vi "Daq.Gui.vi"() -> ()   [LabVIEW 2016]
uses:
  Daq.Gui.Action.ctl
  Drivers/V7310/V7310.Data.Status.State.ctl
  Drivers/V7310/LowLevel/V7310.LaserStatus.ctl
  Drivers/FestoCPX/Station/FestoCPX.Station.ProdPresentGUI.ctl
  Drivers/FestoCPX/Station/FestoCPX.Station.RevolverID.ctl
  Drivers/V7310/LowLevel/V7310.Job.Sets.ctl
  tools/Translator/Translator.Message.ctl
  Drivers/V7310/LowLevel/V7310.Job.Data.ctl
  Station/Station.ValvePosition.ctl
  Station/Station.ProductSlot.ctl
  Drivers/FestoCPX/Station/FestoCPX.Station.ProdArmPosition.ctl
  <vilib>/Utility/miscctls.llb/LVRowAndColumnTypeDef.ctl
  Drivers/FestoCPX/FestoCPX.DO.Data.Fglb.Action.ctl
  tools/CitTemplate/citTemplate.errData.ctl
  tools/EventLog/EventLog.EventSource.ctl
  Station/Station.ProductSuctionGripper.Type.ctl
  tools/Translator/Translator.FormatMessage.vi
  tools/Config/Config.Global.vi
  Global/ApplicationGlobal.vi
  tools/Translator/Translator.Global.vi
  Drivers/FestoCPX/FestoCPX.Global.vi
  Drivers/V7310/LowLevel/V7310.Global.vi
  Sequence/Sequence.Global.vi
  Station/Station.Global.vi
panel:
  out "Run.PeriphsHider 2":bool
  out "Run.PeriphsHider":bool
  out "_loop":i32(ring)=4
  in  "MainTab":enum32{"TABLE", "LASER"}(tab)
  out "ForkID":u8 caption="PopID"
  in  "Btn10":bool caption="Produkt"
  in  "Btn09":bool caption="Blokada"
  in  "Btn07":bool caption="Arm"
  in  "Btn08":bool caption="Arm"
  in  "Btn06":bool caption="Ramię"
  in  "Btn03":bool caption="Table"
  out "RevolverID":T1 caption="MagID"
  in  "Btn17":bool caption="Sucker Slot L B"
  in  "Btn16":bool caption="Sucker Slot L A"
  in  "Btn18":bool caption="Sucker Slot T A"
  in  "Btn19":bool caption="Sucker Slot T B"
  in  "Btn20":bool caption="Sucker Slot R A"
  in  "Btn21":bool caption="Sucker Slot R B"
  in  "Btn22":bool caption="Sucker Slot B A"
  in  "Btn23":bool caption="Sucker Slot B B"
  in  "Btn04":bool caption="Lift"
  in  "Btn15":bool caption="Koniec"
  in  "Btn14":bool caption="Final"
  in  "Btn05":bool caption="Stół"
  out "ProdPresent":T2
  in  "Laser.PrintB":bool
  in  "Laser.Job.SetsB":T3 caption="B"
  out "Laser.JobInUse":string caption="Wybrany program"
  out "Laser.Job.VarDef":string[](array[string]) caption="Zmienne"
  out "EmgFrontDoorSecured":bool caption="Bezp. Blokada Drzwi"
  out "EmgSideDoor":bool caption="Bezp. Drzwi Bok"
  out "EmgFrontDoor":bool caption="Bezp. Drzwi Front"
  out "EmgButton":bool caption="Bezp. Wyłącznik"
  in  "Btn01":bool caption="Bezp."
  in  "Btn02":bool caption="Blokada\nDrzwi"
  in  "Laser.Job.SetsA":T3 caption="A"
  out "Laser.LaserStatusRaw":string caption="Status"
  out "Laser.TS":timestamp caption="Czas"
  out "Laser.Status":T4 caption="Status"
  out "Laser.State":T5=enum."Init" caption="Stan"
  in  "Btn11":bool caption="Interlock"
  in  "Btn13":bool caption="Odsysacz\noparów"
  in  "Btn12":bool caption="Wyzwolenie"
  in  "Job.Variables":string[](array[string]) caption="Wartości"
  out "AirPressureInside":bool caption="Ciśnienie wewnątrz"
  out "AirPressure":bool caption="Ciśnienie zasilania"
  in  "Btn00":bool caption="Powietrze"
  in  "ScanOrder":bool
  in  "ScanProduct":bool
  in  "Laser.PrintA":bool
  in  "DO.Manual":bool caption="Control"
  in  "DO.Buttons":bool[](array[boolean])
  out "DO":i32(listbox)
  out "DI":i32(listbox)=-1
  out "ButtRefs":refnum<vi>[](array[refnum])
  out "delay":u32
  out "exit":bool
  out "Panel":refnum<vi>
  out "action":T6=enum."--- Daq.Gui ---"
  in  "_align":bool
  # "RAW DATA"
  # "TABLE"
  # "EMERGENCY CIRCUIT"
  # "AIR PRESSURE"
  # "SCANNER"
  # "LASER"
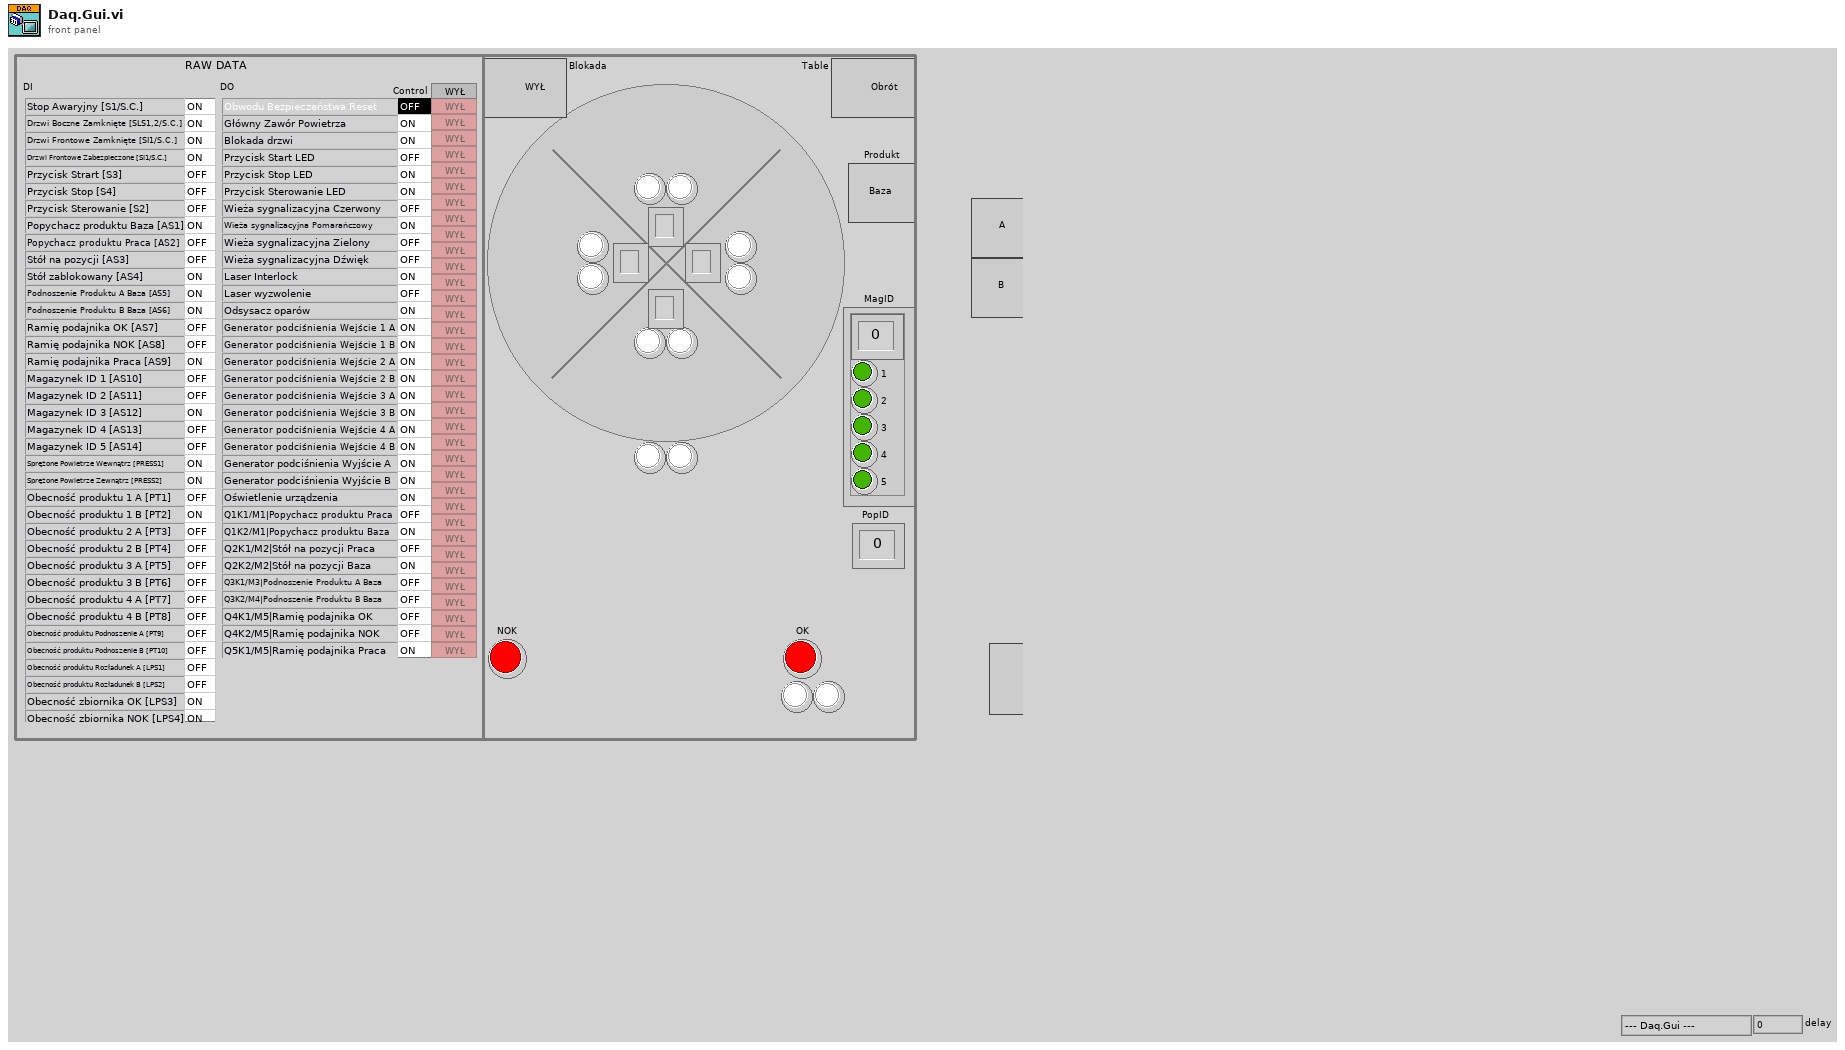
[diagram p1: front panel]
types:
  T1 = typedef "FestoCPX.Station.RevolverID.ctl" = cluster{"ID":u8, "1":bool, "2":bool, "3":bool, "4":bool, "5":bool}
  T2 = typedef "FestoCPX.Station.ProdPresentGUI.ctl" = cluster{"ProdPresentSlotRightA":bool, "ProdPresentSlotRightB":bool, "ProdPresentSlotTopA":bool, "ProdPresentSlotTopB":bool, "ProdPresentSlotLeftA":bool, "ProdPresentSlotLeftB":bool, "ProdPresentSlotBottomA":bool, "ProdPresentSlotBottomB":bool, "SlotNoRight":u8, "SlotNoTop":u8, "SlotNoLeft":u8, "SlotNoBottom":u8, "ProdFinalA":bool, "ProdFinalB":bool, "ProdFinalA 2":bool, "ProdFinalB 2":bool, "ProdContainerOK":bool, "ProdContainerNOK":bool}
  T3 = typedef "V7310.Job.Sets.ctl" = cluster{"X":dbl, "Y":dbl, "Angle":dbl}
  T4 = typedef "V7310.LaserStatus.ctl" = enum16{"-", "FatalError", "Initialize", "KeySwitchOpen", "TimeoutInterlock", "InterlockOpen", "StartUp", "ShutterlockOpen", "Standby", "Ready", "PrepareForMarking", "WaitForTrigger", "Marking"}
  T5 = typedef "V7310.Data.Status.State.ctl" = enum16{"First", "Init", "Msg", "Error", "Abort", "Idle", "Run"}
  T6 = typedef "Daq.Gui.Action.ctl" = enum32{"idle", "constructor", "destructor", "--- Daq.Gui ---", "Open", "Update.IO", "Update.Buttons"}
  T7 = enum8{"Enabled", "Disabled", "Disabled and Grayed Out"}
  T8 = typedef "V7310.Job.Data.ctl" = cluster{"Vars":string[], "Sets":T3}
  T9 = typedef "Translator.Message.ctl" = enum16{"-", "Event confirmed", "Log out", "Log in", "Shutdown", "Cancel", "Start", "Begin time", "End time", "Duration", "Service Mode", "Ignore Results", "Serial Format", "On", "Off", "OK", "NOK", "NOK %s", "Home", "Work", "Close", "Open", "In progress...", "Missing", "Empty", "Hardware failure", "Initial", "Default", "Total", "Out of range", "Free disk space is below 1GB - contact technician", "Error %d >> %s", "Error %d >> %s >> %s", "Msg %d >> %s", "Laser msg %d %s", "Laser cmd error %s %d", "Laser cmd failed %s", "Laser cmd warning %s", "Laser disconnected", "Laser status %s", "Laser already started", "Laser job unkonwn %s", "Laser job missing %s", "Laser job select failure %s", "Unable to start laser printing (%s)", "Unable to stop laser printing (%s)", "Laser marking aborted", "Laser marking timeout", "Unable to reset Laser Interlock (%s)", "Unable to trigger Laser. Laser not ready (%s)", "Laser job '%s' coordinates not configured", "Starting %s", "Quitting %s", "Configured", "Initializing", "Quitting", "Loading", "Loaded %d results", "Loaded %d events", "Running", "Stopped", "Summary", "Laser", "Do you want to continue?", "Do you want to delete the configuration?", "The configuration is being used by an order. Unable to delete!", "Press confirm button", "Station is not based. Do you want to exit?", "Station requires changeover. Do you want to run the test?", "Test options are not set as default. Do you want to continue?", "Formatting of WabcoNo is disabled. Do you want to continue?", "Product not detected. Do you want to continue?", "Product scan failed. Do you want to continue?", "Calibration", "Log out?", "System", "All", "IDLE", "Translating...%s", "Not found", "Alarm %s", "Run", "Skip", "Abort", "Repeat", "Please wait...", "Database disconnected", "Database disconnected - changeover disabled!", "Login to database successful", "Login to database failed: %d; %s", "Unable to check the product status of reference %d - database disconnected", "Unable to set the product status of reference %d - database disconnected", "Variant file backup %s", "Read variant (%s)", "Result", "Station armed!", "Station requires changeover!", "Select reference number...", "EMERGENCY BUTTON - press Control button", "EMERGENCY DOOR - press Control button", "Resetting Emergency...", "Unable to reset safety circuit - Emergency Button pressed", "Unable to reset safety circuit - Emergency Side Door open", "Station not based", "Station based", "Station not empty", "Station basing...", "No order", "Press Start to begin new order", "Scanning new order", "Order NOK. Correct or scan again", "Order OK. Press Accept", "Order ready", "Revolver incorrect", "Fork incorrect", "Revolver missing", "Revolver empty", "Container missing", "Offline results", "Offline statistics", "Updating statistics %.1f %%", "DMC Configurator", "Door open", "Close the front door", "Press start button", "Done. Open the front door", "Running...", "Running...%.1f %%", "Pause %s", "Pause %s. NOK container missing", "Pause %s. OK container missing", "Pause %s. Revolver empty", "Pause %s. Revolver missing", "Pause %s. Revolver incorrect", "Pause %s. Fork missing", "Pause %s. Fork incorrect", "Pause %s. Too many failures", "Pause %s. Unloading failure", "Pause %s. One slot is not working", "Pause %s. Part order is done. Empty OK container", "Pause %s. Unable to move product to slot", "Pause %s. Unable to move back product pusher", "Pause %s. Unable to lift product", "Pause %s. Unable to move back product lifter", "Pause %s. Unable to move product arm to Work", "Pause %s. Unable to move product arm to NOK", "Pause %s. Unable to move product arm to OK", "Pause %s. Unable to unsuck the NOK product", "Pause %s. Unable to drop the NOK product", "Pause %s. Product OK missing", "Pause %s. Unable to unsuck the OK product", "Pause %s. Unable to drop the OK product", "Stopping...", "File '%s' is missing", "File '%s' is broken", "File '%s' is running", "Log file started (%s)", "Log file ended (%s)", "Log file stopped (%s)", "Log file ignored (%s)", "Log file exported (%s)", "Log file export failed (%s)", "Wrong serial number in log file", "Wrong reference number in log file", "Test steps are missing", "%s = %.3f", "Process param '%s' not found in DB", "Process param '%s' wrong order", "Process param '%s' value %.3f out of limits (%.3f; %.3f)", "Step%d param '%s' not found in DB", "Step%d param '%s' wrong order", "Step%d param '%s' value %.3f out of limits (%.3f; %.3f)", "Step%d EV '%s' not found in DB", "Step%d EV '%s' wrong order", "\"%s\" not found in DB", "\"%s\" wrong order", "\"%s\" value %.3f out of limits (%.3f; %.3f)", "\"%s\" not found in software", "Process init (%s)", "Process started", "Process restarted", "Process run", "Process done", "Process done - remove OK container", "Process aborted", "Process aborted at work", "Process aborted at home", "Process error", "Process error at home", "Process error at work", "Process close", "Process pause", "Process continue", "Process door open", "Process door close", "Process pause at slot %s due to %s", "Select plate from the order to process", "Do you want to start the process?", "Do you want to continue the process?", "There is unfinished order. Do you want to put the new order?", "Product %s %d OK", "Product %s %d NOK", "Unable to unload the slot %s. Product missing in the slot", "Unable to unload the slot %s. Product already in the arm", "Unable to accept the product as OK. Product missing in slot %s", "Unable to accept the product as OK. Product could not drop into the container at slot %s", "Unable to accept the product as NOK. Product could not drop into the container at slot %s", "Scan failed. Error %s", "Scan failed. Scanner disconnected", "Scan failed. Wrong Wabco number %d, limit (%d,%d)", "Scan failed. Wrong serial number %d, limit (%d,%d)", "Scan failed. Wrong date %d, limit (%d,%d)", "Scan failed. Wrong product wabco number %d (expected %d)", "Scan failed. Wrong product serial number %d (expected > 0)", "Scan OK %s", "Scan failed. Unable to determine table position (%s)", "Scan failed. Timeout", "Tune failed. Scanner disconnected", "Tune failed. Timeout", "%s = %d", "%s = %d->%d", "Unable to set %s = %.2f - Air Pressure Inside off", "Unable to set digital output '%s' = %d", "Unable to activate air pressure inside - timeout", "Unable to activate air pressure inside - aborted", "Unable to switch on Air Main Valve - Air Pressure Inlet off", "Unable to switch on Air Main Valve - Door open", "Unable to switch off Air Main Valve - timeout", "Unable to switch off Air Main Valve - aborted", "Unable to rotate Table - timeout", "Unable to rotate Table - aborted", "Unable to rotate Table - Product Move not in Home position", "Unable to rotate Table - Air Pressure Inside off", "Unable to rotate Table - Product Lift A not in Home position", "Unable to rotate Table - Product Lift B not in Home position", "Unable to rotate Table - unlock before movement timeout", "Unable to rotate Table - lock after movement timeout", "Unable to move Table Lock to %s position - timeout", "Unable to move Table Lock to %s position - aborted", "Unable to move Table Lock to %s position - Air Pressure Inside off", "Unable to move Table Lock to %s position - Table not in position", "Unable to move Product Lift A to %s position - timeout", "Unable to move Product Lift B to %s position - timeout", "Unable to move Product Lift A to %s position - aborted", "Unable to move Product Lift B to %s position - aborted", "Unable to move Product Lift A to %s position - Air Pressure Inside off", "Unable to move Product Lift B to %s position - Air Pressure Inside off", "Unable to move Product Lift A to %s position - Table not locked", "Unable to move Product Lift B to %s position - Table not locked", "Unable to move Product Lift A to %s position - Product Arm not in Work position", "Unable to move Product Lift B to %s position - Product Arm not in Work position", "Unable to set Product Suction Gripper %s to %s - timeout", "Unable to set Product Suction Gripper %s to %s - aborted", "Unable to set Product Suction Gripper %s to %s - Air Pressure Inside off", "Unable to set Product Suction Gripper %s to %s - Table slot unkown", "Unable to move Product Arm to %s position - timeout", "Unable to move Product Arm to %s position - aborted", "Unable to move Product Arm to %s position - Air Pressure Inside off", "Unable to move Product Arm to %s position - Product Lift A not in Home position", "Unable to move Product Arm to %s position - Product Lift B not in Home position", "Unable to move Product to %s position - timeout", "Unable to move Product to %s position - aborted", "Unable to move Product to %s position - Air Pressure Inside off", "Unable to move Product to %s position - Table not in position"}
  T10 = typedef "Station.ValvePosition.ctl" = enum16{"Home", "Work"}
  T11 = typedef "Station.ProductSlot.ctl" = enum8{"A", "B"}
  T12 = typedef "FestoCPX.Station.ProdArmPosition.ctl" = enum16{"Work", "OK", "NOK"}
  T13 = typedef "LVRowAndColumnTypeDef.ctl" = cluster{"Row":i32, "Column":i32}
  T14 = typedef "FestoCPX.DO.Data.Fglb.Action.ctl" = enum16{"init", "set", "get", "check", "select", "reset"}
  T15 = typedef "EventLog.EventSource.ctl" = enum16{"All", "Gui", "Ref", "File", "Arch", "Seq", "CPX", "DB", "Laser", "Scan.P", "Scan.O"}
  T16 = typedef "citTemplate.errData.ctl" = cluster{"ts":timestamp, "src":T15, "instance":i32, "action":string, "error":errorcluster, "unconfirmed":bool}
  T17 = typedef "Station.ProductSuctionGripper.Type.ctl" = enum8{"Final A", "Final B", "Slot 1 A", "Slot 1 B", "Slot 2 A", "Slot 2 B", "Slot 3 A", "Slot 3 B", "Slot 4 A", "Slot 4 B"}
  T18 = typedef "citTemplate.notifierHandle.ctl" = refnum<notifier>
  T19 = enum32{"Invalid", "Standard", "Closed", "Hidden", "Minimized", "Maximized"}
  T20 = typedef "LVPositionTypeDef.ctl" = cluster{"Left":i32, "Top":i32}
  T21 = typedef "FestoCPX.Data.Sets.ctl" = cluster{"IP":string, "Timeout_ms":i32, "ReconnectPeriod_s":i32, "Config.DI":T22[], "Config.DO":T24[]}
  T22 = typedef "FestoCPX.DI.Sets.ctl" = cluster{"Name":string, "Channel":T23, "Negate":bool}
  T23 = typedef "FestoCPX.DI.ctl" = enum16{"0.0", "0.1", "0.2", "0.3", "0.4", "0.5", "0.6", "0.7", "1.0", "1.1", "1.2", "1.3", "1.4", "1.5", "1.6", "1.7", "2.0", "2.1", "2.2", "2.3", "2.4", "2.5", "2.6", "2.7", "3.0", "3.1", "3.2", "3.3", "3.4", "3.5", "3.6", "3.7", "4.0", "4.1", "4.2", "4.3", "4.4", "4.5", "4.6", "4.7"}
  T24 = typedef "FestoCPX.DO.Sets.ctl" = cluster{"Name":string, "Channel":T25, "Negate":bool, "Default":bool}
  T25 = typedef "FestoCPX.DO.ctl" = enum16{"4.0", "4.1", "4.2", "4.3", "4.4", "4.5", "4.6", "4.7", "5.0", "5.1", "5.2", "5.3", "5.4", "5.5", "5.6", "5.7", "6.0", "6.1", "6.2", "6.3", "6.4", "6.5", "6.6", "6.7", "Q1K1", "Q1K2", "Q2K1", "Q2K2", "Q3K1", "Q3K2", "Q4K1", "Q4K2", "Q5K1", "Q5K2", "Q6K1", "Q6K2"}
  T26 = typedef "Sequence.Data.ctl" = cluster{"BeginTS":timestamp, "EndTS":timestamp, "State":T27, "Status.Work":T28, "Status.Process":T28, "Status.Home":T28, "Status.Wabco":T28, "Status.Client":T28, "BreakReason":T29, "BreakSource":T30, "DoorLock":bool, "Status.Prod":T31[], "UserAction":T35, "UserData":T36, "Error":errorcluster, "Code":T39, "Rotations":i32, "ProdIdx":i32, "ProdDone":T31[], "PrintedSerials-Wabco":i32[], "PrintedSerials-Client":i32[], "Counters-Wabco":T45, "Counters-Client":T45}
  T27 = typedef "Sequence.State.ctl" = enum16{"Init", "Idle", "Home", "Work", "Run", "Pause"}
  T28 = typedef "Sequence.Step.Status.ctl" = enum16{"-", "Pending", "Running", "Skipped", "Passed", "Failed", "Done", "Error", "Aborted", "Stopped"}
  T29 = typedef "Sequence.Test.BreakReason.ctl" = enum16{"-", "NOK container", "OK container", "Rev empty", "Rev missing", "Rev wrong", "Fork missing", "Fork wrong", "NOK limit", "Unload failure", "Single slot", "Part done", "Err: Prod move work", "Err: Prod move home", "Err: Prod lift work", "Err: Prod lift home", "Err: Prod Arm Work", "Err: Prod Arm NOK", "Err: Prod Arm OK", "Err: Prod NOK suck", "Err: Prod NOK drop", "Err: Prod OK missing", "Err: Prod OK suck", "Err: Prod OK drop"}
  T30 = typedef "Sequence.Test.BreakSource.ctl" = enum16{"-", "A", "B", "A/B"}
  T31 = typedef "Sequence.Test.Status.ctl" = cluster{"Slot":T32, "A":T34, "B":T34}
  T32 = typedef "Sequence.Slot.StatusData.ctl" = cluster{"ID":i32, "Unload":T33, "TS":timestamp, "duration":u32}
  T33 = typedef "Sequence.Test.Unload.Status.ctl" = enum16{"init", "check NOK", "check OK", "wait on NOK", "wait on OK", "wait on Unload", "done"}
  T34 = typedef "Sequence.Prod.StatusData.ctl" = cluster{"status":T28, "pause":T29, "present":bool, "printed":bool, "scanned":bool, "tuned":bool, "removed":bool, "OCRignored":bool, "LaserVariables":string[], "Serial":i32, "path":path, "corners":cluster{"X":i32, "Y":i32}[], "verification":u8, "ScanerReadOut":string[]}
  T35 = typedef "Sequence.UserActions.ctl" = cluster{"Stop":bool, "Pause":bool, "Next":bool}
  T36 = typedef "Sequence.UserData.ctl" = cluster{"GuiMode":T37, "Test":T38, "ContinueOrder":bool}
  T37 = typedef "Sequence.MainMode.ctl" = enum16{"Process", "Base", "Order", "Manual", "Logs", "Results", "Stats", "DMC Config"}
  T38 = typedef "MainGui.TestOptions.ctl" = cluster{"IgnoreResults":bool, "IgnoreImages":bool, "ServiceMode":bool}
  T39 = typedef "Sequence.Code.Sets.ctl" = cluster{"Ready":bool, "DoubleOrder":bool, "OrderDone":bool, "AllowSingleSlot":bool, "IgnoreOCR":bool, "ThresholdA":u8, "ThresholdB":u8, "Plate":T40, "ImgPath":path, "Variant":T41}
  T40 = typedef "Sequence.PlateType.ctl" = enum16{"Wabco", "Client"}
  T41 = typedef "Logger.Variant.Sets.ctl" = cluster{"State":T42, "ImgPath":path, "WabcoPlate":string, "WabcoProduct":string, "ClientProduct":string, "ClientPlate":string, "TotalQuantity":u16, "OrderQuantity":u16, "Serial":i32, "Wabco":T43, "Client":T43}
  T42 = typedef "Station.Changeover.State.vi" = enum16{"Init", "Scaning", "NOK", "Wait for ack", "Ready"}
  T43 = typedef "Station.Plate.Properties.ctl" = cluster{"LaserJob":string, "AdditionalTxt":string, "FactoryCode":string, "RevID":u8, "ForkID":u8, "FailuresLimit":u16, "GlobalCnt":i32, "ScannerProgram":u8, "SerialFormat":T44, "CoordA":T3, "CoordB":T3, "DMCconfig":i32, "CVX_Program":u16}
  T44 = typedef "Sequence.Code.SerialFormat.ctl" = enum8{"", "6 dig", "7 dig"}
  T45 = typedef "Sequence.Counters.ctl" = cluster{"Expected":u16, "Done":u16, "OK":u16, "NOK":u16, "NOKlimit":u16, "Part":u16, "PartOK":u16}
  T46 = typedef "V7310.Data.Status.ctl" = cluster{"State":T5, "LaserStatus":T4, "LaserStatusRaw":string, "Ref":refnum<k5>, "RTC TS":timestamp, "Conn TS":timestamp, "Msg":T47[], "JobInUse":string, "Jobs":string[], "Vars":T48[]}
  T47 = typedef "V7310.Message.Data.ctl" = cluster{"ID":i32, "Msg":string}
  T48 = typedef "V7310.Job.Variable.ctl" = cluster{"Name":string, "Value":string}
  T49 = typedef "FestoCPX.Station.ProdPresent.ctl" = cluster{"Slot1":cluster{"A":bool, "B":bool}, "Slot2":cluster{"A":bool, "B":bool}, "Slot3":cluster{"A":bool, "B":bool}, "Slot4":cluster{"A":bool, "B":bool}, "Final":cluster{"A":bool, "B":bool}, "OK":cluster{"A":bool, "B":bool}, "Container":cluster{"OK":bool, "NOK":bool}}
  T50 = typedef "Station.Data.ctl" = cluster{"State":T51, "Seq.State":T27, "Seq.BreakReason":T29, "Seq.BreakSource":T30, "Hw failure":bool, "Unconfirmed":bool, "Station empty":bool, "Home err":bool, "Order done":bool, "DUT present":T49, "EmgState":T52, "Sets":T36, "StatusBits":T53}
  T51 = typedef "Station.State.ctl" = enum16{"Idle", "Ready", "Run", "Stop", "Error", "Home", "Done", "Emg"}
  T52 = typedef "FestoCPX.Station.EmgState.ctl" = cluster{"Button":bool, "SideDoor":bool, "FrontDoor":bool, "DoorSecured":bool}
  T53 = typedef "Station.Home.Status.Bits.ctl" = cluster{"Door Close":bool, "Rev OK":bool, "Fork OK":bool, "Container OK":bool, "Station empty":bool}
  T54 = typedef "FestoCPX.Station.Table.ReadyState.ctl" = cluster{"Air":bool, "Prod Move":bool, "Prod Lift A":bool, "Prod Lift B":bool}
  T55 = typedef "FestoCPX.Station.ProdLift.ReadyState.ctl" = cluster{"Air":bool, "Prod Arm":bool}
  T56 = typedef "FestoCPX.Station.ProdArm.ReadyState.ctl" = cluster{"Air":bool, "Prod Lift A":bool, "Prod Lift B":bool}
  T57 = typedef "FestoCPX.Station.ProdMove.ReadyState.ctl" = cluster{"Air":bool, "Table":bool}
  T58 = typedef "FestoCPX.Station.ProdSuctionGripper.ReadyState.ctl" = cluster{"Air":bool, "TableSlot":bool}
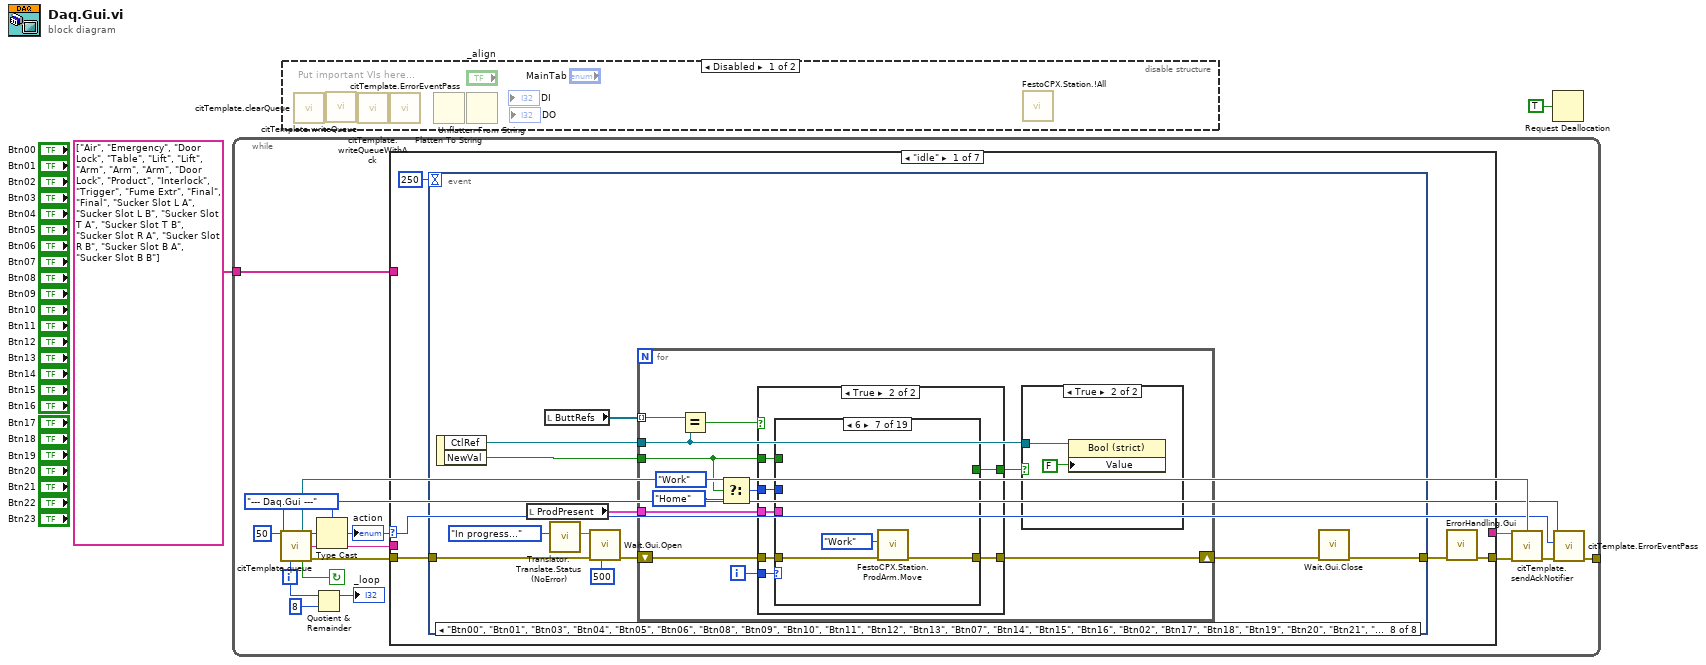
[diagram p0: block diagram]
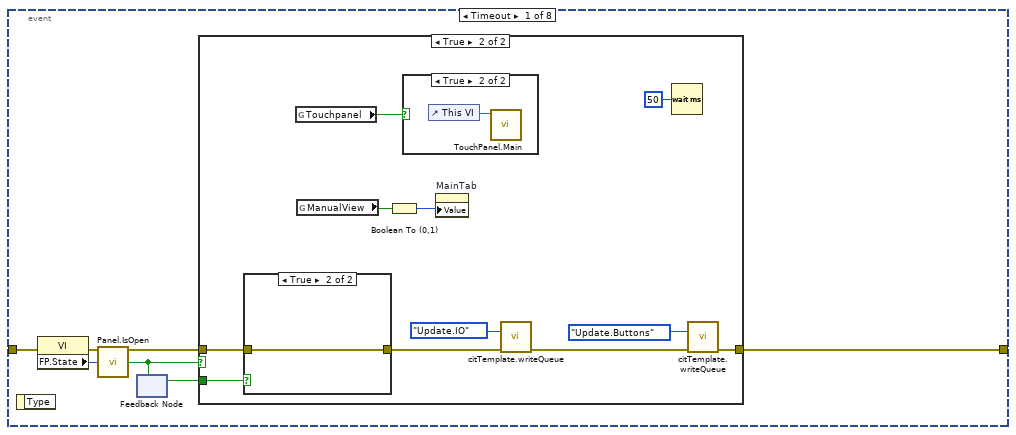
[diagram p3: hidden frame]
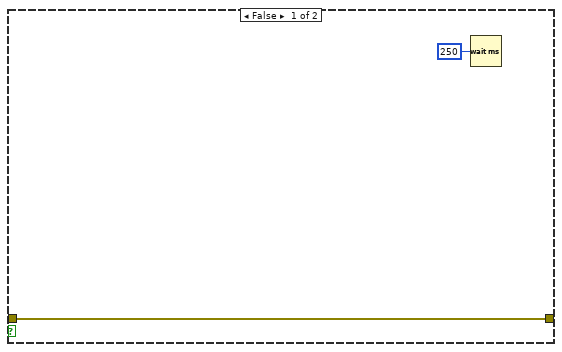
[diagram p4: hidden frame]
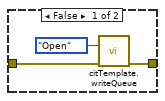
[diagram p5: hidden frame]
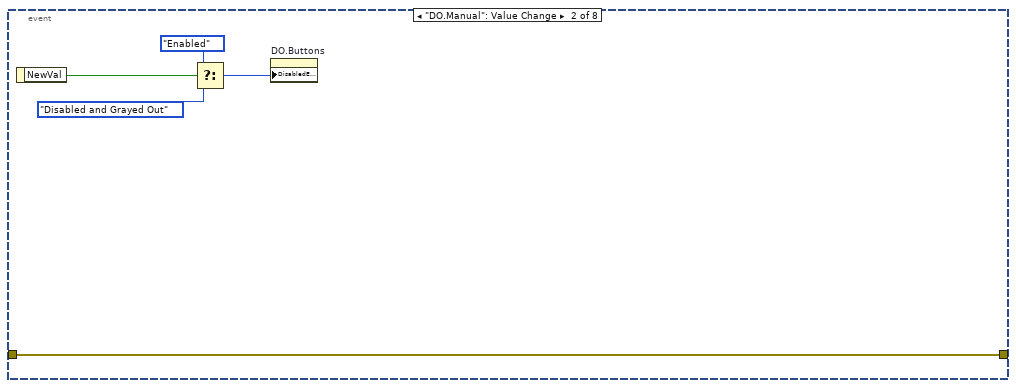
[diagram p7: hidden frame]
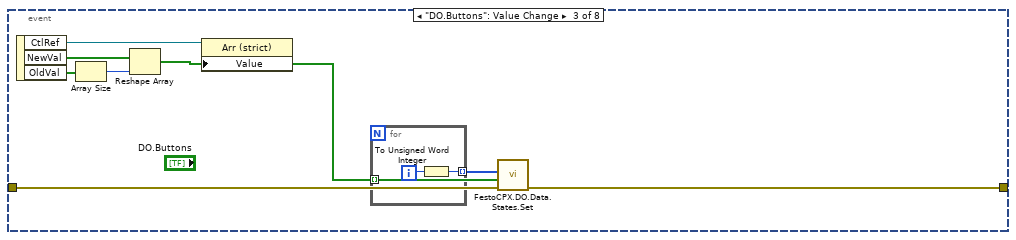
[diagram p8: hidden frame]
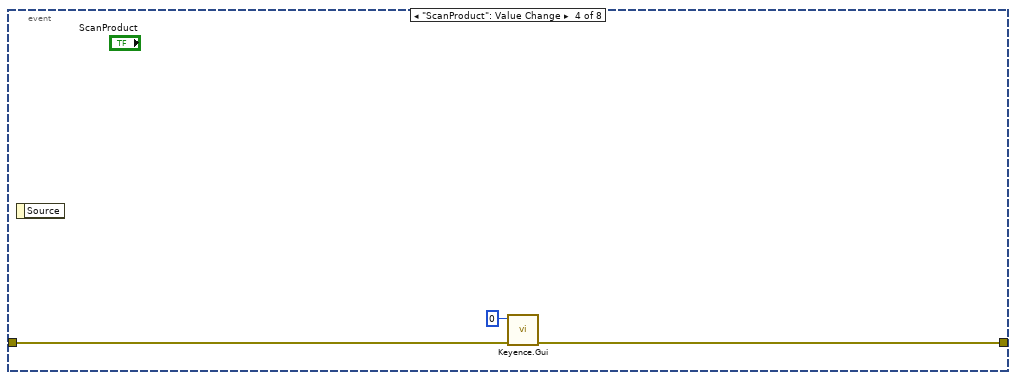
[diagram p9: hidden frame]
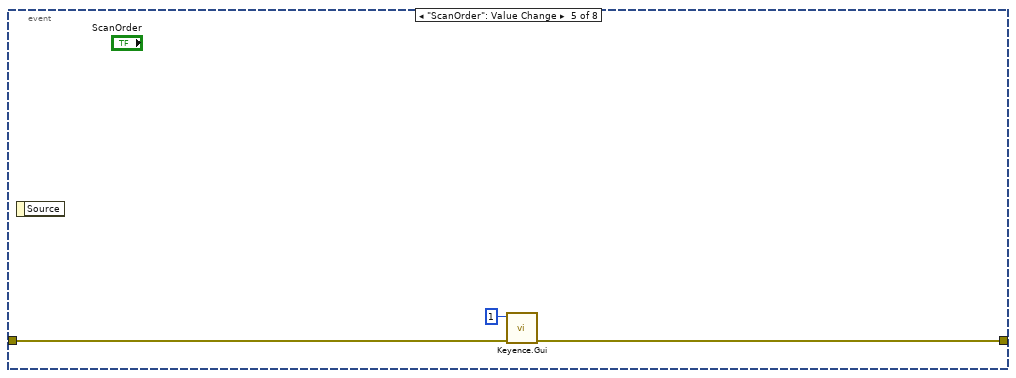
[diagram p10: hidden frame]
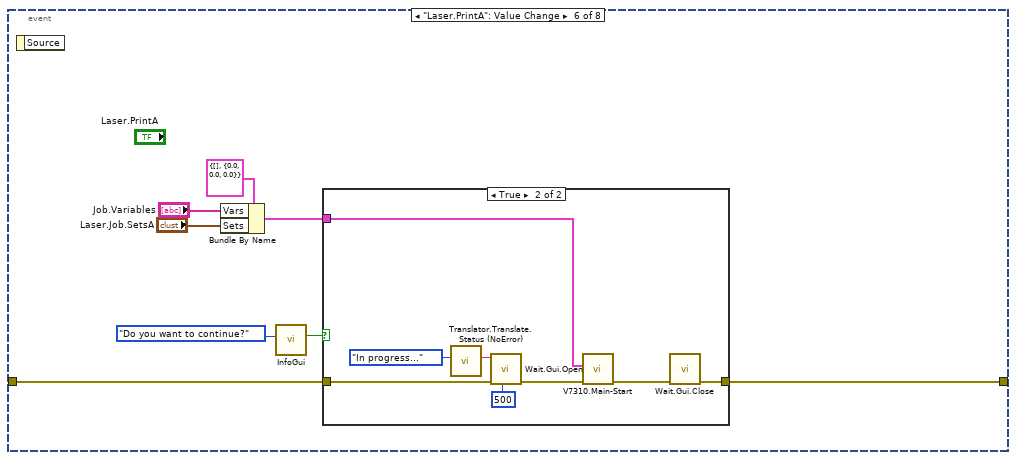
[diagram p11: hidden frame]
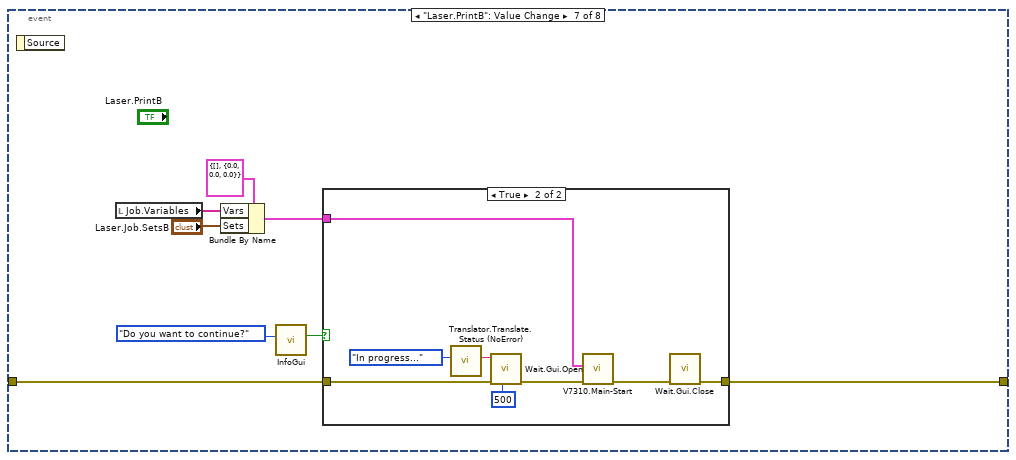
[diagram p13: hidden frame]
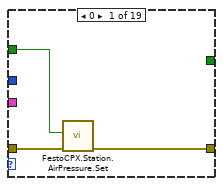
[diagram p17: hidden frame]
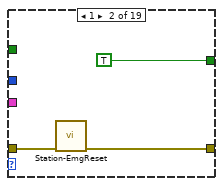
[diagram p18: hidden frame]
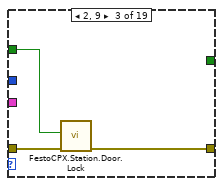
[diagram p19: hidden frame]
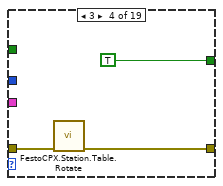
[diagram p20: hidden frame]
diagram:
  n1 = while {
    tunnel: [w7] -> _
    tunnel: string[] ["Air", "Emergency", "Door Lock", "Table", "Lift", "Lift", "Arm", "Arm", "Arm", "Door Lock", "Product", "Interlock", "Trigger", "Fume Extr", "Final", "Final", "Sucker Slot L A", "Sucker Slot L B", "Sucker Slot T A", "Sucker Slot T B", "Sucker Slot R A", "Sucker Slot R B", "Sucker Slot B A", "Sucker Slot B B"] -> [w3]
    i -> [w6]
    stop <- w14 continue-if-true
    w9 = Daq.Gui.Action."--- Daq.Gui ---" ("Action")
    n2 = call "citTemplate.queue.vi"("ms timeout (250 ms)"=50, "event enum"=w9, "iteration (-1)"=w6) -> ("notifierHandle out"=w12:T18, "event out"=w17:u32, "(flatten) data out"=w16:string, "continue"=w14:bool, "error out"=w15:errorcluster)  [unwired: 8 in]
    n3 = Quotient & Remainder(x=w6, y=8) -> (x-y*floor(x/y)=→"_loop":i32)  [unwired: 1 out]
    n4 = Type Cast(type=w9, x=w17) -> (*(type *) &x=w8:T6)
    "action" <- w8
    n5 = case shown="\"idle\"" w8 {
      tunnel: w16 -> [_ _ _ w337 _ _ _]
      tunnel: w15 -> [w20 w233 w328 w336 w360 w379 w471]
      tunnel: [w18 w232 w327 w330 w359 w380 w472] -> w10
      tunnel: [_ _ _ "" _ _ _] -> w11
      tunnel: w3 -> [_ w231 _ _ _ _ _]
      frame "idle" {
        n6 = event shown="[7] \"Btn00\", \"Btn01\", \"Btn03\", \"Btn04\", \"Btn05\", \"Btn06\", \"Btn08\", \"Btn09\", \"Btn10\", \"Btn11\", \"Btn12\", \"Btn13\", \"Btn07\", \"Btn14\", \"Btn15\", \"Btn16\", \"Btn02\", \"Btn17\", \"Btn18\", \"Btn19\", \"Btn20\", \"Btn21\", \"Btn22\", \"Btn23\": Value Change" {
          selector: _ -> [_ _ _ _ _ _ _ _]
          dyn-events: _ -> [_ _ _ _ _ _ _ _]
          timeout: 250 -> [_ _ _ _ _ _ _ _]
          tunnel: [w27 w46 w52 w62 w65 w73 w90 w103] -> w19
          tunnel: w20 -> [w26 w46 w54 w63 w66 w74 w91 w108]
          event Timeout {
            n7 = event-data() -> ()  [unwired: 1 in, 1 out]
            n8 = property class="VI"(error in=w26) -> (error out=w25:errorcluster, "FP.State"=w23:T19)  [unwired: 1 in, 1 out]
            n9 = call "Panel.IsOpen.vi"("FP State"=w23) -> ("Open?"=w22:bool)
            n10 = feedback-in #1(w22) -> ()
            n11 = feedback #1() -> (w24:bool)  [unwired: 1 in]
            n12 = case shown="True" w22 {
              tunnel: [w29 w38] -> w27
              tunnel: w25 -> [w29 w36]
              tunnel: w24 -> [_ w34]
              frame False {
                n13 = Wait (ms)(milliseconds to wait=u32 250) -> ()  [unwired: 1 out]
              }
              frame True {
                n14 = case shown="True" w34 {
                  tunnel: w36 -> [w42 w44]
                  tunnel: [w41 w44] -> w35
                  frame False {
                    n15 = call "citTemplate.writeQueue.vi"("event in (if not connected:all statemachine with data event)"=Daq.Gui.Action."Open" ("Action"), "error in (no error)"=w42) -> ("error out"=w41:errorcluster)  [unwired: 13 in]
                  }
                  frame True {
                  }
                }
                n16 = global read "Config.Global.vi" "Touchpanel"() -> (w37:bool)
                n17 = global read "ApplicationGlobal.vi" "ManualView"() -> (w31:bool)
                n18 = Boolean To (0,1)(Boolean=w31) -> (0, 1=w32:i16)
                n19 = case shown="True" w37 {
                  frame False {
                  }
                  frame True {
                    n20 = control-ref of="This VI"() -> (w45:refnum<vi>)
                    n21 = call "TouchPanel.Main.vi"("VI ref"=w45) -> ()  [unwired: 8 in, 3 out]
                  }
                }
                n22 = property on="MainTab" class="TabCtl (strict)"("Value"=w32) -> ()  [unwired: 2 in, 2 out]
                n23 = call "citTemplate.writeQueue.vi"("event in (if not connected:all statemachine with data event)"=Daq.Gui.Action."Update.IO" ("Action"), "error in (no error)"=w35) -> ("error out"=w39:errorcluster)  [unwired: 13 in]
                n24 = Wait (ms)(milliseconds to wait=u32 50) -> ()  [unwired: 1 out]
                n25 = call "citTemplate.writeQueue.vi"("event in (if not connected:all statemachine with data event)"=Daq.Gui.Action."Update.Buttons" ("Action"), "error in (no error)"=w39) -> ("error out"=w38:errorcluster)  [unwired: 13 in]
              }
            }
          }
          event "DO.Manual": Value Change {
            n26 = event-data() -> ("NewVal"=w50:bool)  [unwired: 1 in]
            n27 = Select(t=T7."Enabled" ("Disabled"), s=w50, f=T7."Disabled and Grayed Out" ("Disabled")) -> (s? t:f=w47:T7)
            n28 = property on="DO.Buttons" class="Arr (strict)"("DisabledEnum"=w47) -> ()  [unwired: 2 in, 2 out]
          }
          event "DO.Buttons": Value Change {
            n29 = event-data() -> ("CtlRef"=w55:refnum<vi>, "NewVal"=w58:bool[], "OldVal"=w57:bool[])  [unwired: 1 in]
            n30 = Array Size(array=w57) -> (size(s)=w56:i32)
            n31 = Reshape Array(w58, w56) -> (w51:bool[])
            n32 = property class="Arr (strict)"(reference=w55, "Value"=w51) -> ()  [unwired: 1 in, 2 out]
            n33 = for {
              tunnel: w51 -> [_] mode=indexing
              tunnel: [w59] -> w53 mode=indexing
              i -> [w60]
              n34 = To Unsigned Word Integer(number=w60) -> (unsigned 16bit integer=w59:u16)
            }
            n35 = call "FestoCPX.DO.Data.States.Set.vi"("error in (no error)"=w54, "State"=w51, "CPX.DO"=w53) -> ("error out"=w52:errorcluster)  [unwired: 8 in]
          }
          event "ScanProduct": Value Change {
            n36 = event-data() -> ()  [unwired: 1 in, 1 out]
            n37 = call "Keyence.Gui.vi"("error in"=w63, "Idx"=0) -> ("error out"=w62:errorcluster)  [unwired: 9 in]
          }
          event "ScanOrder": Value Change {
            n38 = event-data() -> ()  [unwired: 1 in, 1 out]
            n39 = call "Keyence.Gui.vi"("error in"=w66, "Idx"=1) -> ("error out"=w65:errorcluster)  [unwired: 9 in]
          }
          event "Laser.PrintA": Value Change {
            n40 = event-data() -> ()  [unwired: 1 in, 1 out]
            n41 = Bundle By Name(cluster=T8 {"Vars"=[], "Sets"={"X"=0.0, "Y"=0.0, "Angle"=0.0}} ("Job"), "Vars"="Job.Variables", "Sets"="Laser.Job.SetsA") -> (w68:T8)
            n42 = call "InfoGui.vi"("_Msg"=Translator.Message."Do you want to continue?") -> ("ok"=w72:bool)  [unwired: 10 in]
            n43 = case shown="True" w72 {
              tunnel: w74 -> [w75 w79]
              tunnel: [w75 w76] -> w73
              tunnel: w68 -> [_ w83]
              frame False {
              }
              frame True {
                n44 = call "Translator.Translate.Status (NoError).vi"("msg"=Translator.Message."In progress...") -> ("Translated Msg"=w81:string)  [unwired: 10 in]
                n45 = call "Wait.Gui.Open.vi"("Delay at open [ms]"=u32 500, "error in (no error)"=w79, "Msg"=w81) -> ("error out"=w78:errorcluster)  [unwired: 8 in]
                n46 = call "V7310.Main-Start.vi"("error in"=w78, "Job"=w83) -> ("error out"=w77:errorcluster)  [unwired: 8 in, 1 out]
                n47 = call "Wait.Gui.Close.vi"("error in (no error)"=w77) -> ("error out"=w76:errorcluster)  [unwired: 10 in]
              }
            }
          }
          event "Laser.PrintB": Value Change {
            n48 = event-data() -> ()  [unwired: 1 in, 1 out]
            n49 = local read "Job.Variables"() -> (w85:string[])
            n50 = Bundle By Name(cluster=T8 {"Vars"=[], "Sets"={"X"=0.0, "Y"=0.0, "Angle"=0.0}} ("Job"), "Vars"=w85, "Sets"="Laser.Job.SetsB") -> (w86:T8)
            n51 = call "InfoGui.vi"("_Msg"=Translator.Message."Do you want to continue?") -> ("ok"=w89:bool)  [unwired: 10 in]
            n52 = case shown="True" w89 {
              tunnel: w91 -> [w92 w96]
              tunnel: [w92 w93] -> w90
              tunnel: w86 -> [_ w100]
              frame False {
              }
              frame True {
                n53 = call "Translator.Translate.Status (NoError).vi"("msg"=Translator.Message."In progress...") -> ("Translated Msg"=w98:string)  [unwired: 10 in]
                n54 = call "Wait.Gui.Open.vi"("Delay at open [ms]"=u32 500, "error in (no error)"=w96, "Msg"=w98) -> ("error out"=w95:errorcluster)  [unwired: 8 in]
                n55 = call "V7310.Main-Start.vi"("error in"=w95, "Job"=w100) -> ("error out"=w94:errorcluster)  [unwired: 8 in, 1 out]
                n56 = call "Wait.Gui.Close.vi"("error in (no error)"=w94) -> ("error out"=w93:errorcluster)  [unwired: 10 in]
              }
            }
          }
          event "Btn00", "Btn01", "Btn03", "Btn04", "Btn05", "Btn06", "Btn08", "Btn09", "Btn10", "Btn11", "Btn12", "Btn13", "Btn07", "Btn14", "Btn15", "Btn16", "Btn02", "Btn17", "Btn18", "Btn19", "Btn20", "Btn21", "Btn22", "Btn23": Value Change {
            n57 = event-data() -> ("CtlRef"=w110:refnum<vi>, "NewVal"=w111:bool)  [unwired: 1 in]
            n58 = local read "ProdPresent"() -> (w102:T2)
            n59 = local read "ButtRefs"() -> (w109:refnum<vi>[])
            n60 = call "Translator.Translate.Status (NoError).vi"("msg"=Translator.Message."In progress...") -> ("Translated Msg"=w105:string)  [unwired: 10 in]
            n61 = call "Wait.Gui.Open.vi"("Delay at open [ms]"=u32 500, "error in (no error)"=w108, "Msg"=w105) -> ("error out"=w107:errorcluster)  [unwired: 8 in]
            n62 = for {
              tunnel: w111 -> [w116]
              tunnel: w110 -> [w114]
              tunnel: w109 -> [w121] mode=indexing
              shift-right: [w122] -> w104
              shift-left: w107 -> [w123]
              tunnel: w102 -> [w112]
              i -> [w120]
              n63 = Equal?(x=w121, y=w114) -> (x = y?=w119:bool)
              n64 = Select(t=Station.ValvePosition."Work" ("Position"), s=w116, f=Station.ValvePosition."Home" ("Position")) -> (s? t:f=w115:T10)
              n65 = case shown="True" w119 {
                tunnel: w123 -> [w126 w133]
                tunnel: [w126 w132] -> w122
                tunnel: w116 -> [_ w131]
                tunnel: w120 -> [_ w130]
                tunnel: w115 -> [_ w129]
                tunnel: [_ w128] -> w113
                tunnel: w112 -> [_ w127]
                frame False {
                }
                frame True {
                  n66 = case shown="6" w130 {
                    selector: w130 -> [_ _ _ _ _ _ _ _ _ _ _ _ _ w183 w194 w205 w216 w227 _]
                    tunnel: w133 -> [w136 w138 w142 w145 w149 w153 w156 w159 w162 w165 w169 w173 w176 w185 w196 w207 w218 w229 w230]
                    tunnel: [w135 w137 w141 w144 w148 w152 w155 w158 w161 w164 w168 w172 w175 w184 w195 w206 w217 w228 w230] -> w132
                    tunnel: w131 -> [w134 _ w140 _ _ _ _ _ _ _ w167 w171 w174 _ _ _ _ _ _]
                    tunnel: w129 -> [_ _ _ _ w147 w151 _ _ _ w163 _ _ _ w179 w190 w201 w212 w223 _]
                    tunnel: [_ TRUE ("Btn3") _ TRUE ("Btn3") _ _ _ _ _ _ _ _ _ _ _ _ _ _ _] -> w128
                    tunnel: w127 -> [_ _ _ _ _ _ _ _ _ _ _ _ _ _ w187 w198 w209 w220 _]
                    frame 0 {
                      n67 = call "FestoCPX.Station.AirPressure.Set.vi"("error in"=w136, "State"=w134) -> ("error out"=w135:errorcluster)  [unwired: 9 in]
                    }
                    frame 1 {
                      n68 = call "Station-EmgReset.vi"("error in (no error)"=w138) -> ("error out"=w137:errorcluster)  [unwired: 10 in]
                    }
                    frame 2, 9 {
                      n69 = call "FestoCPX.Station.Door.Lock.vi"("error in"=w142, "Lock"=w140) -> ("error out"=w141:errorcluster)  [unwired: 9 in]
                    }
                    frame 3 {
                      n70 = call "FestoCPX.Station.Table.Rotate.vi"("error in"=w145) -> ("error out"=w144:errorcluster)  [unwired: 10 in]
                    }
                    frame 4 {
                      n71 = call "FestoCPX.Station.ProdLift.Move.vi"("error in"=w149, "Position"=w147, "Slot"=Station.ProductSlot."A") -> ("error out"=w148:errorcluster)  [unwired: 8 in]
                    }
                    frame 5 {
                      n72 = call "FestoCPX.Station.ProdLift.Move.vi"("error in"=w153, "Position"=w151, "Slot"=Station.ProductSlot."B") -> ("error out"=w152:errorcluster)  [unwired: 8 in]
                    }
                    frame 6 {
                      n73 = call "FestoCPX.Station.ProdArm.Move.vi"("error in"=w156, "Product Status"=FestoCPX.Station.ProdArmPosition."Work") -> ("error out"=w155:errorcluster)  [unwired: 9 in]
                    }
                    frame 7 {
                      n74 = call "FestoCPX.Station.ProdArm.Move.vi"("error in"=w159, "Product Status"=FestoCPX.Station.ProdArmPosition."OK") -> ("error out"=w158:errorcluster)  [unwired: 9 in]
                    }
                    frame 8 {
                      n75 = call "FestoCPX.Station.ProdArm.Move.vi"("error in"=w162, "Product Status"=FestoCPX.Station.ProdArmPosition."NOK") -> ("error out"=w161:errorcluster)  [unwired: 9 in]
                    }
                    frame 10 {
                      n76 = call "FestoCPX.Station.ProdMove.Move.vi"("error in"=w165, "Position"=w163) -> ("error out"=w164:errorcluster)  [unwired: 8 in, 1 out]
                    }
                    frame 11 {
                      n77 = call "FestoCPX.Station.Laser.Interlock.vi"("error in"=w169, "Wait (T)"=FALSE, "Interlock"=w167) -> ("error out"=w168:errorcluster)  [unwired: 8 in]
                    }
                    frame 12 {
                      n78 = call "FestoCPX.Station.Laser.Trigger.vi"("error in"=w173, "Wait (T)"=FALSE, "Trigger"=w171) -> ("error out"=w172:errorcluster)  [unwired: 7 in, 1 out]
                    }
                    frame 13 {
                      n79 = call "FestoCPX.Station.Laser.FumeExtractUnit.vi"("error in"=w176, "FumeExtractUnit"=w174) -> ("error out"=w175:errorcluster)  [unwired: 9 in]
                    }
                    frame 14, 15 {
                      n80 = Compound Arithmetic op=ADD(w183, invert 14 ("value")) -> (w181:i32)
                      n81 = Quotient & Remainder(x=w181, y=2) -> (x-y*floor(x/y)=w178:i32)  [unwired: 1 out]
                      n82 = To Unsigned Byte Integer(number=w178) -> (unsigned 8bit integer=w177:u8)
                      n83 = call "FestoCPX.Station.ProdSuctionGripper.Set.vi"("error in"=w185, "Position"=w179, "Slot"=w177) -> ("error out"=w184:errorcluster)  [unwired: 7 in, 1 out]
                    }
                    frame 16, 17 {
                      n84 = Unbundle By Name(w187) -> ("SlotNoRight"=w186:u8)
                      n85 = Compound Arithmetic op=ADD(w194, invert 16 ("value")) -> (w192:i32)
                      n86 = Quotient & Remainder(x=w192, y=2) -> (x-y*floor(x/y)=w189:i32)  [unwired: 1 out]
                      n87 = To Unsigned Byte Integer(number=w189) -> (unsigned 8bit integer=w188:u8)
                      n88 = call "FestoCPX.Station.ProdSuctionGripper.Set.vi"("error in"=w196, "Sucker (0: Final)"=w186, "Position"=w190, "Slot"=w188) -> ("error out"=w195:errorcluster)  [unwired: 6 in, 1 out]
                    }
                    frame 18, 19 {
                      n89 = Unbundle By Name(w198) -> ("SlotNoTop"=w197:u8)
                      n90 = Compound Arithmetic op=ADD(w205, invert 18 ("value")) -> (w203:i32)
                      n91 = Quotient & Remainder(x=w203, y=2) -> (x-y*floor(x/y)=w200:i32)  [unwired: 1 out]
                      n92 = To Unsigned Byte Integer(number=w200) -> (unsigned 8bit integer=w199:u8)
                      n93 = call "FestoCPX.Station.ProdSuctionGripper.Set.vi"("error in"=w207, "Sucker (0: Final)"=w197, "Position"=w201, "Slot"=w199) -> ("error out"=w206:errorcluster)  [unwired: 6 in, 1 out]
                    }
                    frame 20, 21 {
                      n94 = Unbundle By Name(w209) -> ("SlotNoLeft"=w208:u8)
                      n95 = Compound Arithmetic op=ADD(w216, invert 18 ("value")) -> (w214:i32)
                      n96 = Quotient & Remainder(x=w214, y=2) -> (x-y*floor(x/y)=w211:i32)  [unwired: 1 out]
                      n97 = To Unsigned Byte Integer(number=w211) -> (unsigned 8bit integer=w210:u8)
                      n98 = call "FestoCPX.Station.ProdSuctionGripper.Set.vi"("error in"=w218, "Sucker (0: Final)"=w208, "Position"=w212, "Slot"=w210) -> ("error out"=w217:errorcluster)  [unwired: 6 in, 1 out]
                    }
                    frame 22, 23 {
                      n99 = Unbundle By Name(w220) -> ("SlotNoBottom"=w219:u8)
                      n100 = Compound Arithmetic op=ADD(w227, invert 18 ("value")) -> (w225:i32)
                      n101 = Quotient & Remainder(x=w225, y=2) -> (x-y*floor(x/y)=w222:i32)  [unwired: 1 out]
                      n102 = To Unsigned Byte Integer(number=w222) -> (unsigned 8bit integer=w221:u8)
                      n103 = call "FestoCPX.Station.ProdSuctionGripper.Set.vi"("error in"=w229, "Sucker (0: Final)"=w219, "Position"=w223, "Slot"=w221) -> ("error out"=w228:errorcluster)  [unwired: 6 in, 1 out]
                    }
                    frame Default {
                    }
                  }
                }
              }
              n104 = case shown="True" w113 {
                tunnel: w114 -> [_ w125]
                frame False {
                }
                frame True {
                  n105 = property on="Property Node" class="Bool (strict)"(reference=w125, "Value"=FALSE ("Btn3")) -> ()  [unwired: 1 in, 2 out]
                }
              }
            }
            n106 = call "Wait.Gui.Close.vi"("error in (no error)"=w104) -> ("error out"=w103:errorcluster)  [unwired: 10 in]
          }
        }
        n107 = call "ErrorHandling.Gui.vi"("error in (no error)"=w19) -> ("error out"=w18:errorcluster)  [unwired: 9 in, 1 out]
      }
      frame "constructor" {
        n108 = stacked-sequence {
          tunnel: w233 -> [_ _ _ w322]
          tunnel: [_ _ _ w321] -> w232
          tunnel: w231 -> [_ _ w294 _]
          frame #0 {
            w237 = u32 0
            n109 = control-ref of="This VI"() -> (w246:refnum<vi>)
            n110 = property on="DO.Manual" class="Bool (strict)"("Value"=FALSE ("DigitalOutputs.ManualControl")) -> ()  [unwired: 2 in, 2 out]
            n111 = property on="DO" class="MCListbox (strict)"("SelColor"=w237) -> (error out=w240:errorcluster)  [unwired: 2 in, 1 out]
            n112 = property class="VI"(reference=w246) -> (reference out=w244:refnum<vi>, error out=w243:errorcluster, "Front Panel"=w247:refnum<vi>, "FP.State"=w241:T19)  [unwired: 1 in]
            n113 = property on="DO" class="MCListbox (strict)"("ActiveCell"=T13 {"Row"=1, "Column"=0} ("Active Cell:Active Cell")) -> (error out=w250:errorcluster, "Height"=w249:u32)  [unwired: 2 in, 1 out]
            n114 = property on="DI" class="MCListbox (strict)"(error in=w240, "SelColor"=w237) -> ()  [unwired: 1 in, 2 out]
            n115 = case shown="\"Standard\", \"Minimized\", \"Maximized\"" w241 {
              tunnel: w244 -> [w255 w259]
              tunnel: w243 -> [w254 w258]
              tunnel: [w255 w257] -> w236
              tunnel: [w254 w256] -> w242
              frame Default {
              }
              frame "Standard", "Minimized", "Maximized" {
                n116 = invoke class="VI" method="FP.Close"(reference=w259, error in=w258) -> (reference out=w257:refnum<vi>, error out=w256:errorcluster)  [unwired: 1 in, 1 out]
              }
            }
            n117 = Compound Arithmetic op=ADD(w249, u32 1 ("value")) -> (w239:u32)
            n118 = property on="OK Button" class="Bool (strict)"(error in=w250, "Height"=w239) -> ()  [unwired: 1 in, 2 out]
            n119 = property on="_align" class="Bool (strict)"() -> (error out=w253:errorcluster, "Position"=w252:T20)  [unwired: 2 in, 1 out]
            n120 = property on="Pane" class="Pane"(error in=w253, "Origin"=w252) -> ()  [unwired: 1 in, 2 out]
            n121 = property class="Pnl"(reference=w247, error in=w242, "DeferPanUpdts"=TRUE ("Defer Panel Updates")) -> (reference out=→"Panel":refnum<vi>)  [unwired: 1 out]
            n122 = global write "ApplicationGlobal.vi" "GuiRef.Daq"(w236) -> ()
            n123 = property on="MainTab" class="TabCtl (strict)"("Value"=enum32{"TABLE", "LASER"}."TABLE" ("MainTab")) -> ()  [unwired: 2 in, 2 out]
          }
          frame #1 {
            w272 = -1 ("Digital Inputs")
            n124 = for {
              N: 50 -> [_]
              i -> [w283]
              w279 = u32 16448250
              n125 = Bundle(w283, 0) -> (w280:cluster{i32, i32})  [unwired: 1 in]
              n126 = property on="DO" class="MCListbox (strict)"("ActiveCell"=w280, "CellBG"=w279) -> (error out=w281:errorcluster)  [unwired: 2 in, 1 out]
              n127 = property on="DI" class="MCListbox (strict)"(error in=w281, "ActiveCell"=w280, "CellBG"=w279) -> ()  [unwired: 1 in, 2 out]
            }
            n128 = property on="DO" class="MCListbox (strict)"("Value"=w272) -> (error out=w273:errorcluster)  [unwired: 2 in, 1 out]
            n129 = property on="DI" class="MCListbox (strict)"(error in=w273, "Value"=w272) -> ()  [unwired: 1 in, 2 out]
            n130 = call "FestoCPX.DO.Data.Fglb.vi"("state (get all)"=FestoCPX.DO.Data.Fglb.Action."get") -> ("error out"=w271:errorcluster, "State out"=w268:bool[])  [unwired: 8 in, 1 out]
            n131 = global read "FestoCPX.Global.vi" "FestoCPX.Sets"() -> (w267:T21)
            n132 = Array Size(array=w268) -> (size(s)=w269:i32)
            n133 = property on="DO.Buttons" class="Arr (strict)"(error in=w271, "Value"=w268, "Number of Rows"=w269, "DisabledEnum"=T7."Disabled and Grayed Out" ("Disabled")) -> ()  [unwired: 1 in, 2 out]
            n134 = Unbundle By Name(w267) -> ("Config.DO"=w262:T24[], "Config.DI"=w263:T22[])
            n135 = Array Size(array=w262) -> (size(s)=w264:i32)
            n136 = for {
              tunnel: w262 -> [w276] mode=indexing
              tunnel: [w275] -> w266 mode=indexing
              n137 = Unbundle By Name(w276) -> ("Name"=w275:string)
            }
            n138 = for {
              tunnel: w263 -> [w278] mode=indexing
              tunnel: [w277] -> w265 mode=indexing
              n139 = Unbundle By Name(w278) -> ("Name"=w277:string)
            }
            n140 = Array Size(array=w263) -> (size(s)=w261:i32)
            n141 = property on="DO" class="MCListbox (strict)"("RowHdrs[]"=w266, "NumRows"=w264) -> ()  [unwired: 2 in, 2 out]
            n142 = property on="DI" class="MCListbox (strict)"("RowHdrs[]"=w265, "NumRows"=w261) -> ()  [unwired: 2 in, 2 out]
          }
          frame #2 {
            n143 = control-ref of="Btn00"() -> (w309:refnum<vi>)
            n144 = control-ref of="Btn01"() -> (w298:refnum<vi>)
            n145 = control-ref of="Btn02"() -> (w308:refnum<vi>)
            n146 = control-ref of="Btn03"() -> (w307:refnum<vi>)
            n147 = control-ref of="Btn04"() -> (w306:refnum<vi>)
            n148 = control-ref of="Btn05"() -> (w305:refnum<vi>)
            n149 = control-ref of="Btn06"() -> (w304:refnum<vi>)
            n150 = control-ref of="Btn07"() -> (w303:refnum<vi>)
            n151 = control-ref of="Btn08"() -> (w302:refnum<vi>)
            n152 = control-ref of="Btn09"() -> (w301:refnum<vi>)
            n153 = control-ref of="Btn10"() -> (w300:refnum<vi>)
            n154 = control-ref of="Btn11"() -> (w299:refnum<vi>)
            n155 = control-ref of="Btn12"() -> (w292:refnum<vi>)
            n156 = control-ref of="Btn13"() -> (w297:refnum<vi>)
            n157 = control-ref of="Btn14"() -> (w296:refnum<vi>)
            n158 = control-ref of="Btn15"() -> (w295:refnum<vi>)
            n159 = control-ref of="Btn16"() -> (w293:refnum<vi>)
            n160 = control-ref of="Btn17"() -> (w286:refnum<vi>)
            n161 = control-ref of="Btn18"() -> (w285:refnum<vi>)
            n162 = control-ref of="Btn19"() -> (w284:refnum<vi>)
            n163 = control-ref of="Btn20"() -> (w290:refnum<vi>)
            n164 = control-ref of="Btn21"() -> (w289:refnum<vi>)
            n165 = control-ref of="Btn22"() -> (w288:refnum<vi>)
            n166 = control-ref of="Btn23"() -> (w287:refnum<vi>)
            n167 = Build Array(w309, w298, w308, w307, w306, w305, w304, w303, w302, w301, w300, w299, w292, w297, w296, w295, w293, w286, w285, w284, w290, w289, w288, w287) -> (w291:refnum<vi>[])
            "ButtRefs" <- w291
            n168 = for {
              tunnel: w291 -> [w318] mode=indexing
              tunnel: w294 -> [w317]
              tunnel: [w316] -> _
              i -> [w310]
              n169 = Index Array(array=w317, index=w310) -> (element=w312:string)
              n170 = Empty String/Path?(string/path=w312) -> (empty?=w315:bool)
              n171 = Not(x=w315) -> (.not. x?=w314:bool)
              n172 = property class="Bool (strict)"(reference=w318, "Caption.Text"=w312, "Blinking"=FALSE, "Visible"=w314, "DisabledEnum"=T7."Enabled" ("Disabled")) -> (error out=w316:errorcluster)  [unwired: 1 in, 1 out]
            }
          }
          frame #3 {
            n173 = local read "Panel"() -> (w320:refnum<vi>)
            n174 = property class="Pnl"(reference=w320, "DeferPanUpdts"=FALSE ("Defer Panel Updates")) -> ()  [unwired: 1 in, 2 out]
            n175 = call "Translator.TranslateThis.Init.vi"("error in"=w322) -> ("error out"=w321:errorcluster)  [unwired: 10 in]
          }
        }
      }
      frame "destructor" {
        n176 = local read "Panel"() -> (w326:refnum<vi>)
        n177 = property class="Pnl"(reference=w326, "DeferPanUpdts"=FALSE ("Defer Panel Updates")) -> (reference out=w324:refnum<vi>, error out=w323:errorcluster)  [unwired: 1 in]
        n178 = Close Reference(reference=w324, error in (no error)=w323) -> ()  [unwired: 1 out]
        n179 = call "Translator.TranslateThis.Exit.vi"("error in"=w328) -> ("error out"=w327:errorcluster)  [unwired: 10 in]
        "exit" <- TRUE ("exit")
      }
      frame "--- Daq.Gui ---" {
        n180 = Unflatten From String(type=T16 {"ts"=timestamp(0 s since 1904-01-01), "src"=enum."All", "instance"=0, "action"="", "error"={"status"=FALSE, "code"=0, "source"=""}, "unconfirmed"=FALSE} ("ErrData"), binary string=w337, error in (no error)=w336) -> (value=w332:T16, error out=w333:errorcluster)  [unwired: 3 out]
        n181 = disable-structure shown="Enabled" {
          disable-tunnel: [w341 w348] -> w330
          disable-tunnel: w333 -> [w339 w351]
          disable-tunnel: w332 -> [w338 w350]
          disable-tunnel: EventLog.EventSource."Gui" ("Event source") -> [_ w349]
          frame Disabled {
            n182 = To Variant(anything=w338) -> (Variant=w340:variant)
            n183 = feedback #2(w340) -> (w343:variant)
            n184 = feedback-in #2(w340) -> ()
            n185 = Not Equal?(x=w343, y=w340) -> (x != y?=w342:bool)
            n186 = case shown="True" w342 {
              tunnel: [w344 w347] -> w341
              tunnel: w339 -> [w344 w345]
              tunnel: w338 -> [_ w346]
              frame False {
              }
              frame True {
                n187 = call "ErrorHandling.Gui.vi"("error in (no error)"=w345, "~ErrData"=w346) -> ("error out"=w347:errorcluster)  [unwired: 8 in, 1 out]
              }
            }
          }
          frame Enabled {
            n188 = call "ErrorHandling.Fglb.Add.vi"("Event source"=w349, "error in (no error)"=w351, "Error in"=w350) -> ("error out"=w352:errorcluster, "changed?"=w353:bool)  [unwired: 7 in]
            n189 = case shown="True" w353 {
              tunnel: [w354 w358] -> w348
              tunnel: w350 -> [_ w357]
              tunnel: w352 -> [w354 w356]
              tunnel: w349 -> [_ w355]
              frame False {
              }
              frame True {
                n190 = call "EventLog.New(error).vi"("Source (All)"=w355, "error in"=w356, "ErrData"=w357) -> ("error out"=w358:errorcluster)  [unwired: 8 in]
              }
            }
          }
        }
      }
      frame "Open" {
        n191 = stacked-sequence {
          tunnel: w360 -> [_ w374]
          tunnel: [_ w373] -> w359
          frame #0 {
            n192 = global read "Sequence.Global.vi" "SeqData"() -> (w364:T26)
            n193 = global read "V7310.Global.vi" "Laser.Status"() -> (w369:T46)
            n194 = Unbundle By Name(w364) -> ("Code.Variant.Wabco"=w363:T43)  [unwired: 1 out]
            n195 = Unbundle By Name(w369) -> ("Vars"=w368:T48[], "JobInUse"=w365:string)
            n196 = for {
              tunnel: w368 -> [w372] mode=indexing
              tunnel: [w371] -> w367 mode=indexing
              tunnel: [w370] -> w366 mode=indexing
              n197 = Unbundle(w372) -> ("Name"=w371:string, "Value"=w370:string)
            }
            "Laser.Job.VarDef" <- w367
            n198 = Unbundle By Name(w363) -> ("CoordA"=w362:T3, "CoordB"=w361:T3)
            n199 = local write "Laser.Job.SetsA"(w362) -> ()
            n200 = local write "Laser.Job.SetsB"(w361) -> ()
            n201 = local write "Job.Variables"(w366) -> ()
            n202 = local write "Laser.JobInUse"(w365) -> ()
          }
          frame #1 {
            n203 = disable-structure shown="Enabled" {
              disable-tunnel: w374 -> [w376 w378]
              disable-tunnel: [w375 w378] -> w373
              frame Disabled {
                n204 = global read "ApplicationGlobal.vi" "SettingsPath"() -> (w377:path)
                n205 = call "V7310.File.Write.vi"("error in"=w376, "SettingsPath"=w377) -> ("error out"=w375:errorcluster)  [unwired: 9 in]
              }
              frame Enabled {
              }
            }
          }
        }
      }
      frame "Update.IO" {
        n206 = stacked-sequence {
          seq-local: [_ w383 _ _ _ _ _] -> [_ _ _ _ _ w456 _]
          tunnel: [_ _ w385 _ _ _ _] -> w380
          tunnel: w379 -> [_ _ w385 _ _ _ _]
          frame #0 {
            n207 = local read "Panel"() -> (w382:refnum<vi>)
            n208 = property class="Pnl"(reference=w382, "DeferPanUpdts"=TRUE ("Defer Panel Updates")) -> ()  [unwired: 1 in, 2 out]
          }
          frame #1 {
            n209 = Tick Count (ms)() -> (millisecond timer value=w383:u32)
          }
          frame #2 {
            n210 = call "FestoCPX.DO.Data.Fglb.vi"("state (get all)"=FestoCPX.DO.Data.Fglb.Action."get") -> ("State out"=w392:bool[])  [unwired: 8 in, 2 out]
            n211 = for {
              tunnel: w392 -> [w402] mode=indexing
              tunnel: [w403] -> w395 mode=indexing
              i -> [w406]
              n212 = Select(t=u32 8454016, s=w402, f=u32 16744576) -> (s? t:f=w409:u32)
              n213 = Bundle(w406, 0) -> (w407:cluster{i32, i32})  [unwired: 1 in]
              n214 = property on="DO" class="MCListbox (strict)"("ActiveCell"=w407, "CellBG"=w409) -> ()  [unwired: 2 in, 2 out]
              n215 = Select(t="ON" ("string"), s=w402, f="OFF" ("string")) -> (s? t:f=w403:string)
            }
            n216 = case shown="False" "DO.Manual" {
              tunnel: w392 -> [w401 _]
              frame False {
                n217 = property on="DO.Buttons" class="Arr (strict)"("Value"=w401) -> ()  [unwired: 2 in, 2 out]
              }
              frame True {
              }
            }
            n218 = Build Array(w395) -> (w394:string[][])
            n219 = call "FestoCPX.Station.ProdPresent.Check.vi"() -> ("error out"=w387:errorcluster, "Prod Present"=w389:T49)  [unwired: 6 in, 4 out]
            n220 = Transpose 2D Array(2D array=w394) -> (transposed array=w396:string[][])
            n221 = call "FestoCPX.Station.ProdPresent.Group.vi"("error in"=w387, "Prod Present"=w389) -> ("Prod Present GUI"=→"ProdPresent":T2)  [unwired: 8 in, 1 out]
            n222 = property on="DO" class="MCListbox (strict)"("ItemNames"=w396) -> ()  [unwired: 2 in, 2 out]
            n223 = call "FestoCPX.DI.Data.Fglb.vi"() -> ("error out"=w398:errorcluster, "data out"=w399:bool[])  [unwired: 7 in, 3 out]
            n224 = for {
              tunnel: w399 -> [w412] mode=indexing
              tunnel: [w417] -> w400 mode=indexing
              tunnel: w398 -> [w423]
              tunnel: [w422] -> _
              i -> [w418]
              n225 = Select(t="ON" ("string"), s=w412, f="OFF" ("string")) -> (s? t:f=w417:string)
              n226 = Select(t=u32 8454016, s=w412, f=u32 16744576) -> (s? t:f=w419:u32)
              n227 = Bundle(w418, 0) -> (w420:cluster{i32, i32})  [unwired: 1 in]
              n228 = property on="DI" class="MCListbox (strict)"(error in=w423, "ActiveCell"=w420, "CellBG"=w419) -> (error out=w422:errorcluster)  [unwired: 1 in, 1 out]
            }
            n229 = call "FestoCPX.Station.Revolver.GetID.vi"() -> ("ForkID"=→"ForkID":u8, "RevID"=→"RevolverID":T1)  [unwired: 9 in, 1 out]
            n230 = Build Array(w400) -> (w397:string[][])
            n231 = Transpose 2D Array(2D array=w397) -> (transposed array=w390:string[][])
            n232 = property on="DI" class="MCListbox (strict)"("ItemNames"=w390) -> ()  [unwired: 2 in, 2 out]
          }
          frame #3 {
            n233 = global read "Station.Global.vi" "Station"() -> (w428:T50)
            n234 = global read "V7310.Global.vi" "Laser.Status"() -> (w436:T46)
            n235 = Unbundle By Name(w428) -> ("State"=w427:T51)
            n236 = Unbundle By Name(w436) -> ("State"=→"Laser.State":T5, "LaserStatus"=w432:T4, "RTC TS"=→"Laser.TS":timestamp, "LaserStatusRaw"=→"Laser.LaserStatusRaw":string, "JobInUse"=→"Laser.JobInUse":string, "Vars"=w426:T48[])  [unwired: 1 out]
            "Laser.Status" <- w432
            n237 = for {
              tunnel: w426 -> [w439] mode=indexing
              tunnel: [w438] -> w425 mode=indexing
              tunnel: [w437] -> w424 mode=indexing
              n238 = Unbundle(w439) -> ("Name"=w438:string, "Value"=w437:string)
            }
            n239 = local write "Laser.Job.VarDef"(w425) -> ()
            n240 = case shown="\"Run\"" w427 {
              tunnel: w424 -> [_ w440]
              frame Default {
              }
              frame "Run" {
                n241 = local write "Job.Variables"(w440) -> ()
              }
            }
            n242 = case shown="\"Standby\", \"Ready\"" w432 {
              tunnel: [w441 T7."Enabled" ("Disabled") T7."Disabled and Grayed Out" ("Disabled")] -> w429
              tunnel: [w441 T7."Disabled and Grayed Out" ("Disabled") T7."Enabled" ("Disabled")] -> _
              frame Default {
                w441 = T7."Disabled and Grayed Out" ("Disabled")
              }
              frame "Standby", "Ready" {
              }
              frame "Marking" {
              }
            }
            n243 = property on="Laser.PrintA" class="Bool"("DisabledEnum"=w429) -> (error out=w430:errorcluster)  [unwired: 2 in, 1 out]
            n244 = property on="Laser.PrintB" class="Bool"(error in=w430, "DisabledEnum"=w429) -> ()  [unwired: 1 in, 2 out]
          }
          frame #4 {
            n245 = global read "Station.Global.vi" "Station"() -> (w451:T50)
            n246 = global read "ApplicationGlobal.vi" "Unlock"() -> (w447:bool)
            n247 = Unbundle By Name(w451) -> ("State"=w450:T51)
            n248 = Not(x=w447) -> (.not. x?=w446:bool)
            n249 = case shown="\"Run\"" w450 {
              tunnel: [T7."Enabled" ("Disabled") T7."Disabled and Grayed Out" ("Disabled")] -> _
              tunnel: [w452 TRUE ("Parker.STO1")] -> w448
              tunnel: w446 -> [w452 _]
              frame Default {
              }
              frame "Run" {
              }
            }
            n250 = property on="Run.PeriphsHider" class="Bool (strict)"("Visible"=w448) -> (error out=w449:errorcluster)  [unwired: 2 in, 1 out]
            n251 = property on="Run.PeriphsHider 2" class="Bool (strict)"(error in=w449, "Visible"=w448) -> ()  [unwired: 1 in, 2 out]
          }
          frame #5 {
            n252 = Tick Count (ms)() -> (millisecond timer value=w458:u32)
            n253 = Subtract(x=w458, y=w456) -> (x-y=→"delay":u32)
          }
          frame #6 {
            n254 = local read "Panel"() -> (w460:refnum<vi>)
            n255 = property class="Pnl"(reference=w460, "DeferPanUpdts"=FALSE ("Defer Panel Updates")) -> ()  [unwired: 1 in, 2 out]
          }
        }
      }
      frame "Update.Buttons" {
        n256 = call "FestoCPX.Station.ProdSuctionGripper.Check.vi"() -> ("error out"=w462:errorcluster, "States"=w463:bool[])  [unwired: 10 in]
        n257 = local read "ButtRefs"() -> (w474:refnum<vi>[])
        n258 = call "FestoCPX.Station.ProdSuctionGripper.Group.vi"("error in"=w462, "States in"=w463) -> ("States out"=w461:bool[])  [unwired: 8 in, 1 out]
        n259 = call "FestoCPX.Station.ProdArm.Check.vi"() -> ("NOK"=w464:bool, "OK"=w465:bool, "Work"=w466:bool)  [unwired: 7 in, 2 out]
        n260 = call "FestoCPX.Station.Laser.Check.vi"("error in"=w471) -> ("error out"=w470:errorcluster, "fume extract unit"=w467:bool, "trigger"=w468:bool, "interlock"=w469:bool)  [unwired: 7 in]
        n261 = stacked-sequence {
          tunnel: w470 -> [_ w486 _ _]
          tunnel: w474 -> [_ w485 _ _]
          tunnel: [_ w484 _ _] -> w473
          tunnel: w469 -> [_ w483 _ _]
          tunnel: w468 -> [_ w482 _ _]
          tunnel: w467 -> [_ w481 _ _]
          tunnel: w466 -> [_ w480 _ _]
          tunnel: w465 -> [_ w479 _ _]
          tunnel: w464 -> [_ w478 _ _]
          tunnel: w461 -> [_ w477 _ _]
          frame #0 {
            n262 = local read "Panel"() -> (w475:refnum<vi>)
            n263 = property class="Pnl"(reference=w475, "DeferPanUpdts"=TRUE ("Defer Panel Updates")) -> ()  [unwired: 1 in, 2 out]
          }
          frame #1 {
            n264 = for {
              tunnel: w486 -> [w497]
              tunnel: [w495] -> w484 mode=indexing
              tunnel: w485 -> [w494] mode=indexing
              workers-P: _ -> [_]
              tunnel: w483 -> [w493]
              tunnel: w482 -> [w492]
              tunnel: w481 -> [w491]
              tunnel: w480 -> [w490]
              tunnel: w479 -> [w489]
              tunnel: w478 -> [w488]
              tunnel: w477 -> [w487]
              i -> [w496]
              n265 = case shown="4" w496 {
                selector: w496 -> [_ _ _ _ _ _ w607 _ w650 w674 _]
                tunnel: w497 -> [w503 w511 w520 w522 w542 w572 w601 w625 w648 w672 w678]
                tunnel: w494 -> [w504 _ w518 w526 w535 w565 w608 w618 w651 w673 _]
                tunnel: [w502 w510 w519 w523 w541 w571 w600 w624 w648 w671 w678] -> w495
                tunnel: w493 -> [_ _ _ _ _ _ _ _ w647 _ _]
                tunnel: w492 -> [_ _ _ _ _ _ _ _ w646 _ _]
                tunnel: w491 -> [_ _ _ _ _ _ _ _ w645 _ _]
                tunnel: w490 -> [_ _ _ _ _ _ w605 _ _ _ _]
                tunnel: w489 -> [_ _ _ _ _ _ w604 _ _ _ _]
                tunnel: w488 -> [_ _ _ _ _ _ w603 _ _ _ _]
                tunnel: w487 -> [_ _ _ _ _ _ _ _ _ w675 _]
                frame 0 {
                  n266 = call "FestoCPX.Station.AirPressure.Check.vi"("error in"=w503) -> ("error out"=w502:errorcluster, "Main Air Valve"=w500:bool, "Air pressure Inside"=w498:bool, "Air pressure Inlet"=→"AirPressure":bool)  [unwired: 7 in]
                  "AirPressureInside" <- w498
                  n267 = Not Equal?(x=w498, y=w500) -> (x != y?=w501:bool)
                  n268 = property on="Property Node" class="Bool (strict)"(reference=w504, "Value"=w500, "Blinking"=w501) -> ()  [unwired: 1 in, 2 out]
                }
                frame 1 {
                  n269 = call "FestoCPX.Station.Emg.Check.vi"("error in"=w511) -> ("error out"=w510:errorcluster, "Emg"=w509:T52)  [unwired: 8 in, 1 out]
                  n270 = Unbundle By Name(w509) -> ("Button"=→"EmgButton":bool, "FrontDoor"=→"EmgFrontDoor":bool, "SideDoor"=→"EmgSideDoor":bool, "DoorSecured"=→"EmgFrontDoorSecured":bool)
                }
                frame 2, 9 {
                  n271 = call "FestoCPX.Station.Door.Check.vi"("error in"=w520) -> ("error out"=w519:errorcluster, "Close"=w516:bool, "Lock"=w517:bool)  [unwired: 8 in]
                  n272 = Compound Arithmetic op=OR(w517, w516) -> (w515:bool)
                  n273 = Select(t=T7."Enabled" ("Disabled"), s=w515, f=T7."Disabled and Grayed Out" ("Disabled")) -> (s? t:f=w512:T7)
                  n274 = property on="Property Node" class="Bool (strict)"(reference=w518, "Value"=w517, "DisabledEnum"=w512) -> ()  [unwired: 1 in, 2 out]
                }
                frame 3 {
                  n275 = call "FestoCPX.Station.Table.Ready.vi"("Log (T)"=FALSE, "error in"=w522) -> ("error out"=w523:errorcluster, "Ready state"=w528:T54)  [unwired: 8 in]
                  n276 = Cluster To Array(cluster=w528) -> (array=w529:bool[])
                  n277 = Or Array Elements(Boolean array=w529) -> (logical OR=w521:bool)
                  n278 = Select(t=T7."Disabled and Grayed Out" ("Disabled"), s=w521, f=T7."Enabled" ("Disabled")) -> (s? t:f=w524:T7)
                  n279 = property on="Property Node" class="Bool (strict)"(reference=w526, "Value"=FALSE, "DisabledEnum"=w524) -> ()  [unwired: 1 in, 2 out]
                }
                frame 4 {
                  w532 = Station.ProductSlot."A" ("Slot")
                  n280 = call "FestoCPX.Station.ProdLift.CheckSlot.vi"("error in"=w542, "Slot"=w532) -> ("error out"=w548:errorcluster, "Work"=w544:bool, "Home"=w533:bool)  [unwired: 7 in]
                  n281 = Compound Arithmetic op=OR(w533, w544) -> (w543:bool)
                  n282 = case shown="False" w543 {
                    tunnel: w544 -> [_ w558]
                    tunnel: [w555 w561] -> w539
                    tunnel: w535 -> [w557 w560]
                    tunnel: [w556 w559] -> w538
                    tunnel: [w554 w558] -> w536
                    frame False {
                      n283 = property on="Property Node" class="Bool (strict)"(reference=w557) -> (reference out=w556:refnum<vi>, error out=w555:errorcluster, "Value"=w554:bool)  [unwired: 1 in]
                    }
                    frame True {
                      n284 = property on="Property Node" class="Bool (strict)"(reference=w560, "Value"=w558) -> (reference out=w559:refnum<vi>, error out=w561:errorcluster)  [unwired: 1 in]
                    }
                  }
                  n285 = Not(x=w543) -> (.not. x?=w537:bool)
                  n286 = Select(t=Station.ValvePosition."Home" ("Position"), s=w536, f=Station.ValvePosition."Work" ("Position")) -> (s? t:f=w540:T10)
                  n287 = call "FestoCPX.Station.ProdLift.Ready.vi"("Log (T)"=FALSE, "error in"=w548, "Position"=w540, "Slot"=w532) -> ("error out"=w541:errorcluster, "Ready state"=w549:T55)  [unwired: 6 in]
                  n288 = Cluster To Array(cluster=w549) -> (array=w550:bool[])
                  n289 = Or Array Elements(Boolean array=w550) -> (logical OR=w534:bool)
                  n290 = Select(t=T7."Disabled and Grayed Out" ("Disabled"), s=w534, f=T7."Enabled" ("Disabled")) -> (s? t:f=w552:T7)
                  n291 = property on="Property Node" class="Bool (strict)"(reference=w538, error in=w539, "Blinking"=w537, "DisabledEnum"=w552) -> ()  [unwired: 2 out]
                }
                frame 5 {
                  w562 = Station.ProductSlot."B" ("Slot")
                  n292 = call "FestoCPX.Station.ProdLift.CheckSlot.vi"("error in"=w572, "Slot"=w562) -> ("error out"=w578:errorcluster, "Work"=w574:bool, "Home"=w563:bool)  [unwired: 7 in]
                  n293 = Compound Arithmetic op=OR(w563, w574) -> (w573:bool)
                  n294 = case shown="False" w573 {
                    tunnel: w574 -> [_ w588]
                    tunnel: [w585 w591] -> w569
                    tunnel: w565 -> [w587 w590]
                    tunnel: [w586 w589] -> w568
                    tunnel: [w584 w588] -> w566
                    frame False {
                      n295 = property on="Property Node" class="Bool (strict)"(reference=w587) -> (reference out=w586:refnum<vi>, error out=w585:errorcluster, "Value"=w584:bool)  [unwired: 1 in]
                    }
                    frame True {
                      n296 = property on="Property Node" class="Bool (strict)"(reference=w590, "Value"=w588) -> (reference out=w589:refnum<vi>, error out=w591:errorcluster)  [unwired: 1 in]
                    }
                  }
                  n297 = Not(x=w573) -> (.not. x?=w567:bool)
                  n298 = Select(t=Station.ValvePosition."Home" ("Position"), s=w566, f=Station.ValvePosition."Work" ("Position")) -> (s? t:f=w570:T10)
                  n299 = call "FestoCPX.Station.ProdLift.Ready.vi"("Log (T)"=FALSE, "error in"=w578, "Position"=w570, "Slot"=w562) -> ("error out"=w571:errorcluster, "Ready state"=w579:T55)  [unwired: 6 in]
                  n300 = Cluster To Array(cluster=w579) -> (array=w580:bool[])
                  n301 = Or Array Elements(Boolean array=w580) -> (logical OR=w564:bool)
                  n302 = Select(t=T7."Disabled and Grayed Out" ("Disabled"), s=w564, f=T7."Enabled" ("Disabled")) -> (s? t:f=w582:T7)
                  n303 = property on="Property Node" class="Bool (strict)"(reference=w568, error in=w569, "Blinking"=w567, "DisabledEnum"=w582) -> ()  [unwired: 2 out]
                }
                frame 6..8 {
                  n304 = case shown="8" w607 {
                    tunnel: w605 -> [_ w611 _ _]
                    tunnel: w604 -> [_ _ w613 _]
                    tunnel: w603 -> [_ _ _ w615]
                    tunnel: [_ w611 w613 w615] -> w606
                    tunnel: [FestoCPX.Station.ProdArmPosition."Work" ("Position") FestoCPX.Station.ProdArmPosition."Work" ("Position") FestoCPX.Station.ProdArmPosition."OK" ("Position") FestoCPX.Station.ProdArmPosition."NOK" ("Position")] -> w593
                    frame Default {
                    }
                    frame 6 {
                    }
                    frame 7 {
                    }
                    frame 8 {
                    }
                  }
                  n305 = Compound Arithmetic op=OR(w605, w604, w603) -> (invert w602:bool)
                  n306 = call "FestoCPX.Station.ProdArm.Ready.vi"("Log (T)"=FALSE, "error in"=w601, "Position"=w593) -> ("error out"=w600:errorcluster, "Ready state"=w597:T56)  [unwired: 7 in]
                  n307 = Cluster To Array(cluster=w597) -> (array=w598:bool[])
                  n308 = Or Array Elements(Boolean array=w598) -> (logical OR=w596:bool)
                  n309 = Select(t=T7."Disabled and Grayed Out" ("Disabled"), s=w596, f=T7."Enabled" ("Disabled")) -> (s? t:f=w594:T7)
                  n310 = property on="Property Node" class="Bool (strict)"(reference=w608, "Value"=w606, "Blinking"=w602, "DisabledEnum"=w594) -> ()  [unwired: 1 in, 2 out]
                }
                frame 10 {
                  n311 = call "FestoCPX.Station.ProdMove.Check.vi"("error in"=w625) -> ("error out"=w631:errorcluster, "Work"=w627:bool, "Home"=w616:bool)  [unwired: 8 in]
                  n312 = Compound Arithmetic op=OR(w616, w627) -> (w626:bool)
                  n313 = case shown="False" w626 {
                    tunnel: w627 -> [_ w641]
                    tunnel: [w638 w644] -> w622
                    tunnel: w618 -> [w640 w643]
                    tunnel: [w639 w642] -> w621
                    tunnel: [w637 w641] -> w619
                    frame False {
                      n314 = property on="Property Node" class="Bool (strict)"(reference=w640) -> (reference out=w639:refnum<vi>, error out=w638:errorcluster, "Value"=w637:bool)  [unwired: 1 in]
                    }
                    frame True {
                      n315 = property on="Property Node" class="Bool (strict)"(reference=w643, "Value"=w641) -> (reference out=w642:refnum<vi>, error out=w644:errorcluster)  [unwired: 1 in]
                    }
                  }
                  n316 = Not(x=w626) -> (.not. x?=w620:bool)
                  n317 = Select(t=Station.ValvePosition."Home" ("Position"), s=w619, f=Station.ValvePosition."Work" ("Position")) -> (s? t:f=w623:T10)
                  n318 = call "FestoCPX.Station.ProdMove.Ready.vi"("Log (T)"=FALSE, "error in"=w631, "Position"=w623) -> ("error out"=w624:errorcluster, "Ready state"=w632:T57)  [unwired: 7 in]
                  n319 = Cluster To Array(cluster=w632) -> (array=w633:bool[])
                  n320 = Or Array Elements(Boolean array=w633) -> (logical OR=w617:bool)
                  n321 = Select(t=T7."Disabled and Grayed Out" ("Disabled"), s=w617, f=T7."Enabled" ("Disabled")) -> (s? t:f=w635:T7)
                  n322 = property on="Property Node" class="Bool (strict)"(reference=w621, error in=w622, "Blinking"=w620, "DisabledEnum"=w635) -> ()  [unwired: 2 out]
                }
                frame 11..13 {
                  n323 = case shown="Default" w650 {
                    tunnel: w647 -> [_ w652 _ _]
                    tunnel: w646 -> [_ _ w653 _]
                    tunnel: w645 -> [_ _ _ w654]
                    tunnel: [_ w652 w653 w654] -> w649
                    frame Default {
                    }
                    frame 11 {
                    }
                    frame 12 {
                    }
                    frame 13 {
                    }
                  }
                  n324 = property on="Property Node" class="Bool (strict)"(reference=w651, "Value"=w649) -> ()  [unwired: 1 in, 2 out]
                }
                frame 14..23 {
                  n325 = Compound Arithmetic op=ADD(w674, invert 14 ("y")) -> (w656:i32)
                  n326 = To Unsigned Byte Integer(number=w656) -> (unsigned 8bit integer=w658:u8)
                  n327 = Index Array(array=w675, index=w656) -> (element=w661:bool)
                  n328 = Equal To 0?(x=w656) -> (x = 0?=w655:bool)
                  n329 = Compound Arithmetic op=ADD(w658, Station.ProductSuctionGripper.Type."Final A" ("Type")) -> (w659:u8)
                  n330 = Select(t=Station.ValvePosition."Home" ("Position"), s=w661, f=Station.ValvePosition."Work" ("Position")) -> (s? t:f=w660:T10)
                  n331 = call "FestoCPX.Station.ProdSuctionGripper.Ready.vi"("Log (T)"=FALSE, "error in"=w672, "Position"=w660, "Type"=w659) -> ("error out"=w671:errorcluster, "Ready state"=w664:T58)  [unwired: 6 in]
                  n332 = Cluster To Array(cluster=w664) -> (array=w665:bool[])
                  n333 = Or Array Elements(Boolean array=w665) -> (logical OR=w667:bool)
                  n334 = Select(t=T7."Disabled and Grayed Out" ("Disabled"), s=w667, f=T7."Enabled" ("Disabled")) -> (s? t:f=w657:T7)
                  n335 = property on="Property Node" class="Bool (strict)"(reference=w673, "Value"=w661, "DisabledEnum"=w657) -> ()  [unwired: 1 in, 2 out]
                  n336 = case shown="True" w655 {
                    tunnel: w657 -> [_ w677]
                    frame False {
                    }
                    frame True {
                      n337 = property on="ProdPresent" class="Clust (strict)"("DisabledEnum"=w677) -> ()  [unwired: 2 in, 2 out]
                    }
                  }
                }
                frame Default {
                }
              }
            }
          }
          frame #2 {
          }
          frame #3 {
            n338 = local read "Panel"() -> (w679:refnum<vi>)
            n339 = property class="Pnl"(reference=w679, "DeferPanUpdts"=FALSE ("Defer Panel Updates")) -> ()  [unwired: 1 in, 2 out]
          }
        }
        n340 = Merge Errors(w473) -> (w472:errorcluster)
      }
    }
    n341 = call "citTemplate.sendAckNotifier.vi"("notification data"=w11, "notifierHandle in"=w12, "error in"=w10) -> ()  [unwired: 13 in]
    n342 = call "citTemplate.ErrorEventPass.vi"("error in"=w10, "action of error"=w8, "event in"=w9) -> ("error out"=w7:errorcluster)  [unwired: 8 in]
  }
  n343 = disable-structure shown="Disabled" {
    frame Disabled {
      # "Put important VIs here..."
      n344 = call "citTemplate.clearQueue.vi"() -> ()  [unwired: 14 in, 2 out]
      n345 = call "citTemplate.writeQueue.vi"() -> ()  [unwired: 15 in, 1 out]
      n346 = call "citTemplate.writeQueueWithAck.vi"() -> ()  [unwired: 13 in, 3 out]
      n347 = call "citTemplate.ErrorEventPass.vi"() -> ()  [unwired: 11 in, 1 out]
      n348 = Flatten To String() -> ()  [unwired: 4 in, 3 out]
      n349 = Unflatten From String() -> ()  [unwired: 5 in, 3 out]
      n350 = call "FestoCPX.Station.!All.vi"() -> ()  [unwired: 12 in]
    }
    frame Enabled {
    }
  }
  n351 = Request Deallocation(TRUE ("flag")) -> ()
